vi "Main.vi"() -> ()   [LabVIEW 2020, in "RxnRover.lvlib"]
doc: "Use this template to build a simple state machine design pattern. Each state executes code and determines which state to transition to."
uses:
  RxnRover.lvlib
  RxnRover/Type Definitions/Data.ctl
  <userlib>/RxnRover/DynamicReentrant/src/Type Defs/Message.ctl
  RxnRover/Plugin Servers/Controller Array/Controller Array.lvclass
  RxnRover/Plugin Manager/Plugin Details.ctl
  RxnRover/Plugin Servers/Controller/Controller Type.ctl
  RxnRover/Plugin Manager/Plugin Types.ctl
  RxnRover/Plugin Manager/Config Error.ctl
  RxnRover/Type Definitions/New Parameters.ctl
  RxnRover/Plugin Servers/Parameter to Hardware Map/Parameter to Hardware Map.lvclass
  RxnRover/Experiment/Experiment File/Experiment File Cluster.ctl
  RxnRover/Plugin Servers/Controller/Minimal Controller Cluster.ctl
  RxnRover/Plugin Servers/Parameter to Hardware Map/Minimal Map.ctl
  RxnRover/Plugin Servers/Parameter to Hardware Map/Minimal Pair Cluster.ctl
  RxnRover/User Preferences/User Preferences File.lvclass
  RxnRover/events/Process Stopped Cluster.ctl
  RxnRover/Type Definitions/Error Levels.ctl
  RxnRover/Plugin Servers/Controller/Generic Plugin.lvclass/Generic Plugin.ctl
  RxnRover/Plugin Servers/Controller Array/Controller Array.lvclass/Controller Array.ctl
  RxnRover/Plugin Servers/Controller Array/Searchable Properties.ctl
  RxnRover/Plugin Servers/Generic Optimizer/Generic Optimizer.lvclass
  RxnRover/Sub VIs/Message Queue/Enqueue Message (Single).vi
  <vilib>/Utility/error.llb/Error Cluster From Error Code.vi
  RxnRover/Plugin Servers/Controller/Generic Plugin.lvclass
  <vilib>/ErrorRing/Error Ring.xnode
  <userlib>/RxnRover/DynamicReentrant/Dynamic Reentrant.lvlib
  RxnRover/Sub VIs/Message Queue/test Message Queue.lvlib
  RxnRover/Experiment/Experiment Manager/Experiment Manager.lvlib
  RxnRover/Experiment/Experiment File/Experiment File.lvlib
  RxnRover/Plugin Manager/Plugin Manager.lvlib
  RxnRover/logging/logging.lvlib
panel:
  in  "Stop Hardware Run Btn":bool
  in  "Start Hardware Run Btn":bool
  in  "Exit":bool
  in  "Stop Analyzer Btn":bool
  in  "Load Analyzer Btn":bool
  in  "Stop Optimizer Btn":bool
  in  "Load Optimizer Btn":bool
  in  "Stop Controller Btn":bool
  in  "Load Control Panel":bool
  in  "View an Analyzer":u16(ring) items=["None"]
  in  "Reorder Analyzers":bool
  in  "Auto Param Passing":bool=TRUE
  in  "Reassign Parameters":bool
  in  "Reject Suggestions":bool
  in  "Accept Suggestions":bool
  out "# of controllers cached":i32
  in  "Select a Plugin":u16(ring) items=["None", "Mock Temperature Controller Control Panel.lvlib:Main.vi:4140001"]
  out "# of analyzers cached":i32
  out "# of optimizers cached":i32
  out "# of plugins cached":i32
  in  "List of Running Plugins":i32(listbox)=-1
  out "Status Bar Text":string
  # "Manual Control"
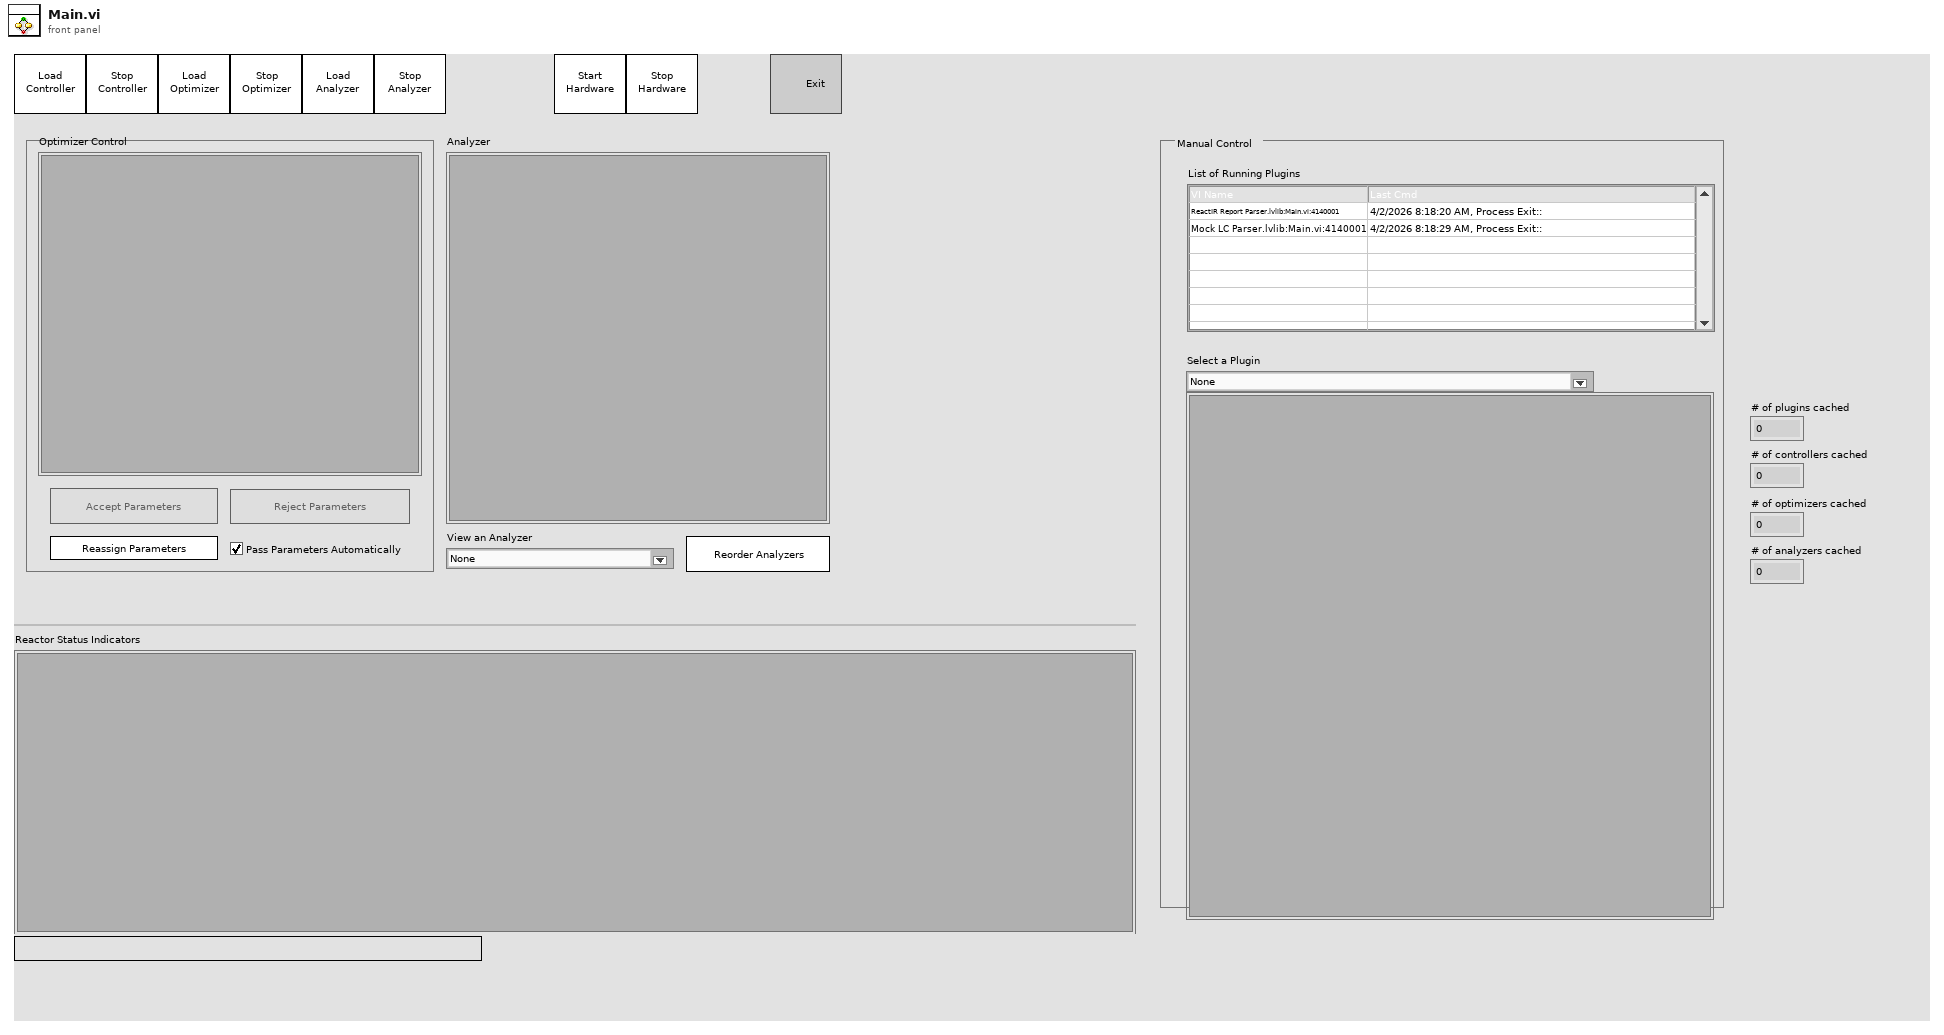
[diagram p1: front panel]
types:
  T1 = enum32{"Invalid", "Standard", "Closed", "Hidden", "Minimized", "Maximized"}
  T2 = typedef "RxnRover.lvlib/Data.ctl" = cluster{"Visible Hardware VI":string, "Current Message":T3, "Message History":string[][], "Hardware":cluster{"Process Cache":refnum<class "Controller Array.lvclass">, "Plugins":T4[]}, "Optimizers":cluster{"Process Cache":refnum<class "Controller Array.lvclass">, "Plugins":T4[], "First parameteres?":bool, "New Parameters":T8}, "Parameter to Hardware Map":refnum<class "Parameter to Hardware Map.lvclass">, "Analyzers":cluster{"Process Cache":refnum<class "Controller Array.lvclass">, "Plugins":T4[]}, "Log Directory":path, "Auto Pass Parameters":bool, "Experiment":cluster{"Name":string, "File Path":path, "File Extension":string, "File Cluster":T9}, "Main VI Queue":refnum<queue>, "Process Queue References":refnum<queue>[], "Message Queue":refnum<queue>, "User Preferences File":refnum<class "User Preferences File.lvclass">}
  T3 = typedef "Dynamic Reentrant.lvlib/Message.ctl" = cluster{"Source":string, "Destination":string, "Time Stamp":timestamp, "Command":string, "Data":variant}
  T4 = typedef "RxnRover.lvlib/Plugin Manager.lvlib/Plugin Details.ctl" = cluster{"Plugin Name":string, "Controller Type":T5, "Control Panel Path":path, "Plugin Type":T6, "Config Errors":T7[]}
  T5 = typedef "RxnRover.lvlib/Generic Plugin.lvclass/Controller Type.ctl" = enum16{"Invalid", "Temperature Controller", "Pump Controller", "Syringe Pump", "Generic Optimizer", "LC Parser", "Passive Hardware"}
  T6 = typedef "RxnRover.lvlib/Plugin Manager.lvlib/Plugin Types.ctl" = enum16{"Invalid", "Optimizer", "Analyzer", "Hardware"}
  T7 = typedef "RxnRover.lvlib/Plugin Manager.lvlib/Config Error.ctl" = cluster{"Error?":bool, "Message":string}
  T8 = typedef "RxnRover.lvlib/New Parameters.ctl" = cluster{"Time Stamp":timestamp, "Names":string[], "Values":variant[]}
  T9 = typedef "RxnRover.lvlib/Experiment File.lvlib/Experiment File Cluster.ctl" = cluster{"Hardware List":T10[], "Optimizer List":T10[], "Analyzer List":T10[], "Parameter to Hardware Map":T11}
  T10 = typedef "RxnRover.lvlib/Generic Plugin.lvclass/Minimal Controller Cluster.ctl" = cluster{"Name":string, "Controller Type":string, "Control Panel Path":string, "Resource":string}
  T11 = typedef "RxnRover.lvlib/Parameter to Hardware Map.lvclass/Minimal Map.ctl" = T12[]
  T12 = typedef "RxnRover.lvlib/Parameter to Hardware Map.lvclass/Minimal Pair Cluster.ctl" = cluster{"key":string, "values":T10[]}
  T13 = typedef "RxnRover.lvlib/Error Levels.ctl" = enum16{"Fatal", "Warning"}
  T14 = typedef "RxnRover.lvlib/Controller Array.lvclass/Searchable Properties.ctl" = enum16{"Name", "Controller Type"}
  T15 = enum8{"Enabled", "Disabled", "Disabled and Grayed Out"}
  T16 = typedef "RxnRover.lvlib/Parameter to Hardware Map.lvclass/Pair.ctl" = cluster{"key":string, "values":refnum<class "Generic Plugin.lvclass">[]}
  T17 = typedef "RxnRover.lvlib/Process Stopped Cluster.ctl" = cluster{"Name":string, "Type":enum16{"Hardware", "Optimizer", "Analyzer"}}
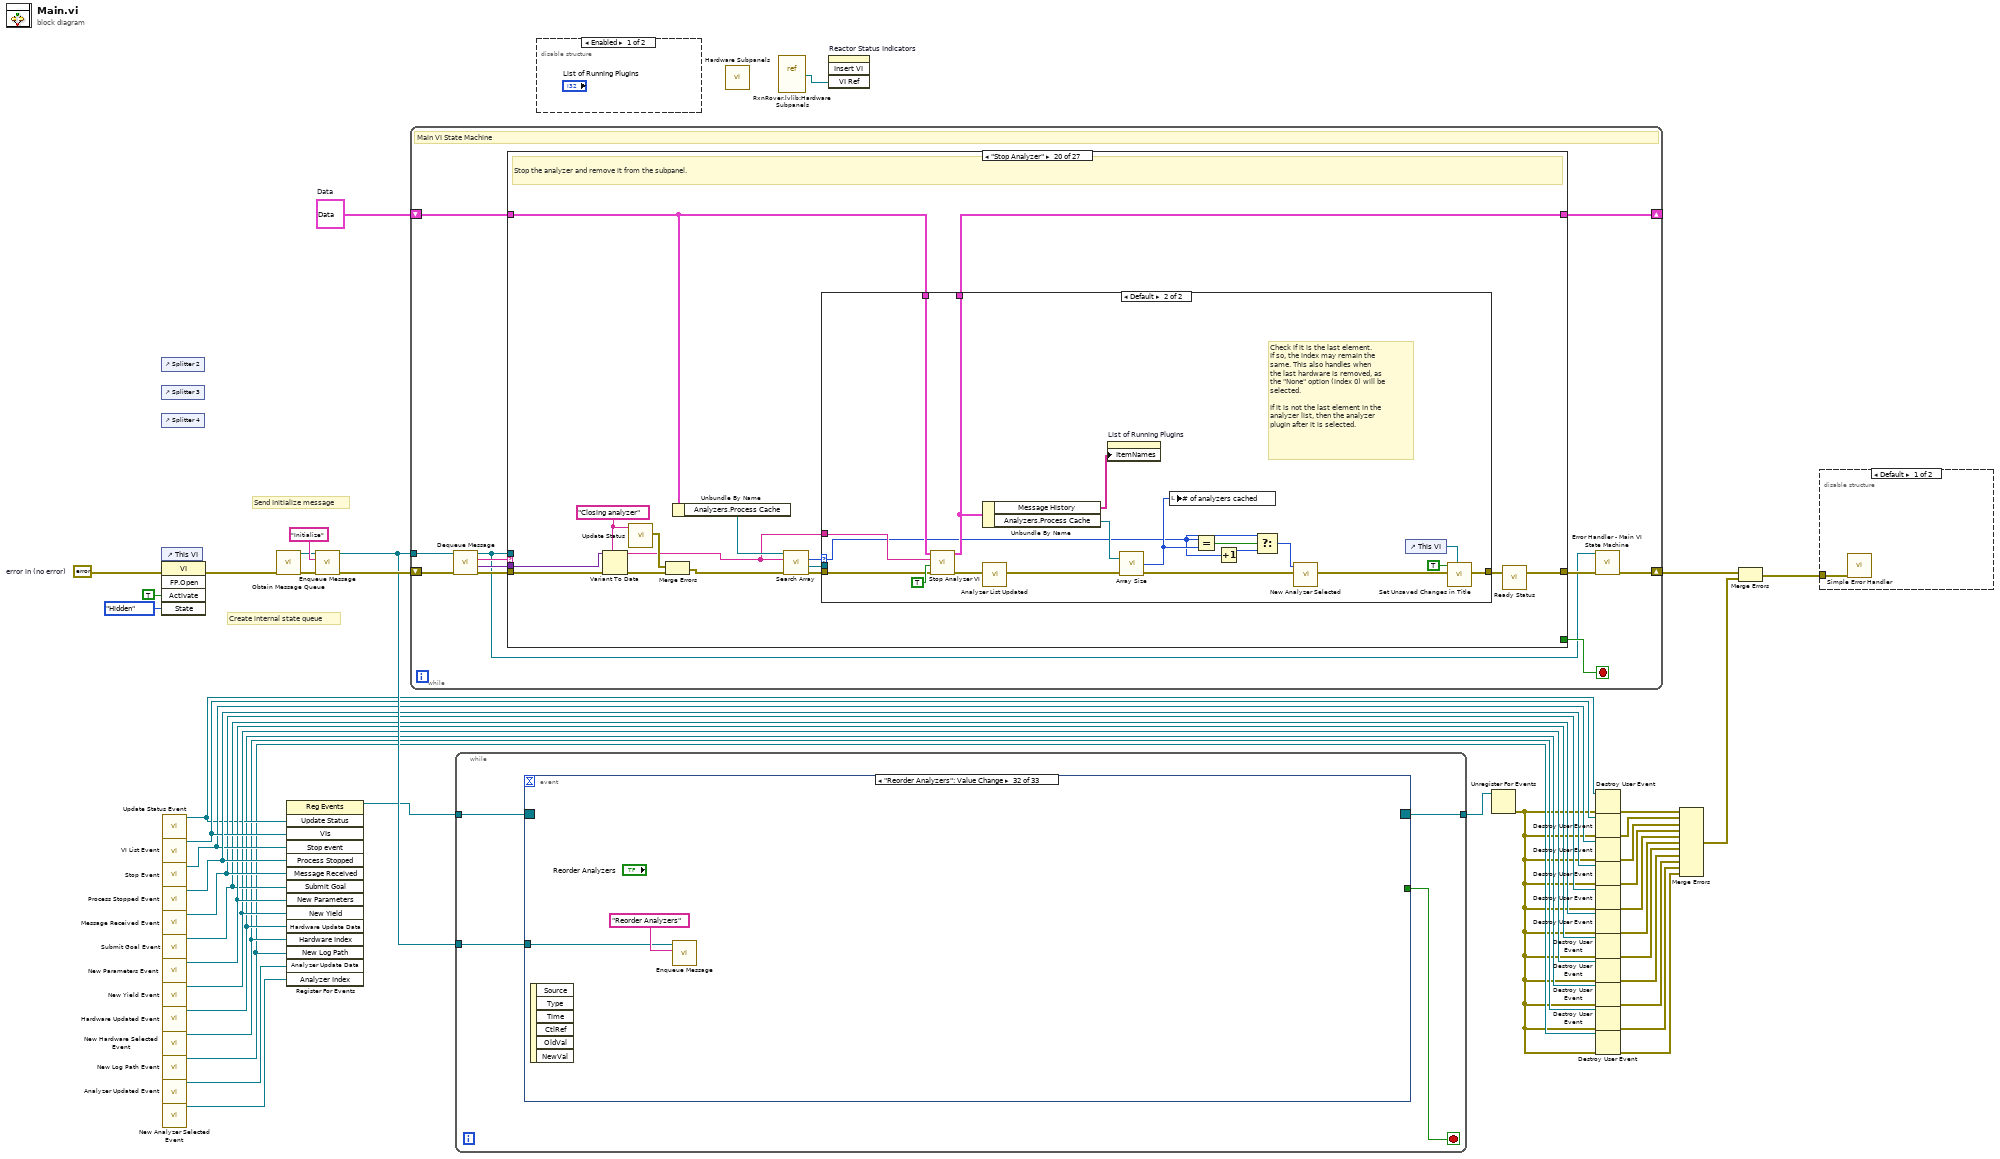
[diagram p0: block diagram]
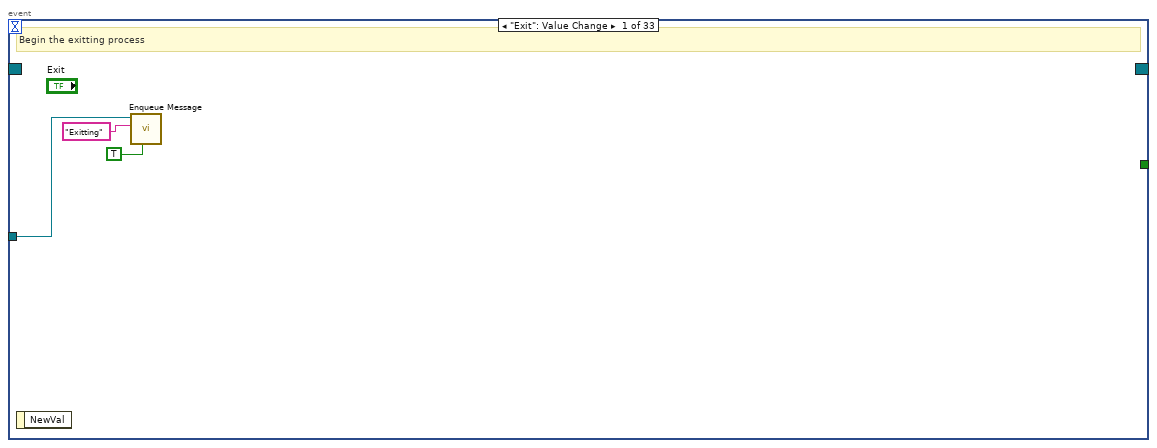
[diagram p2: hidden frame]
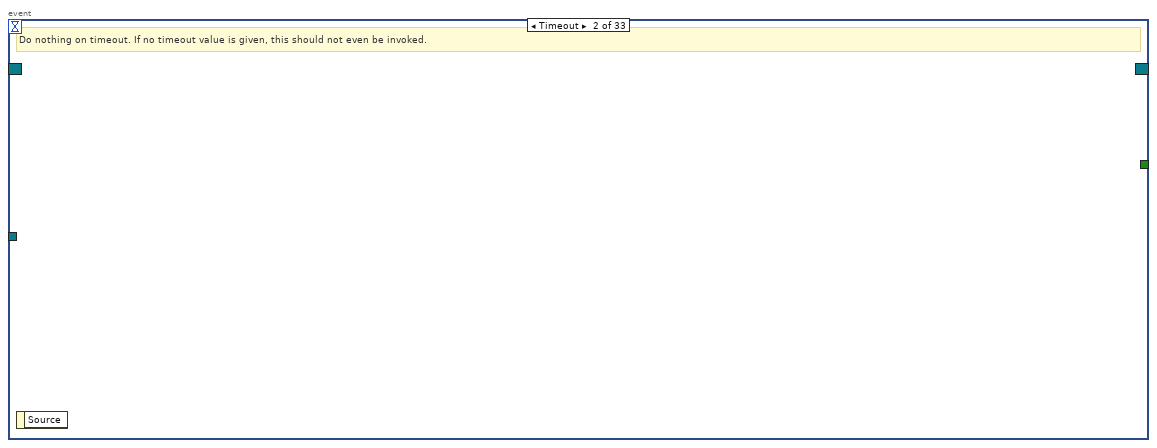
[diagram p3: hidden frame]
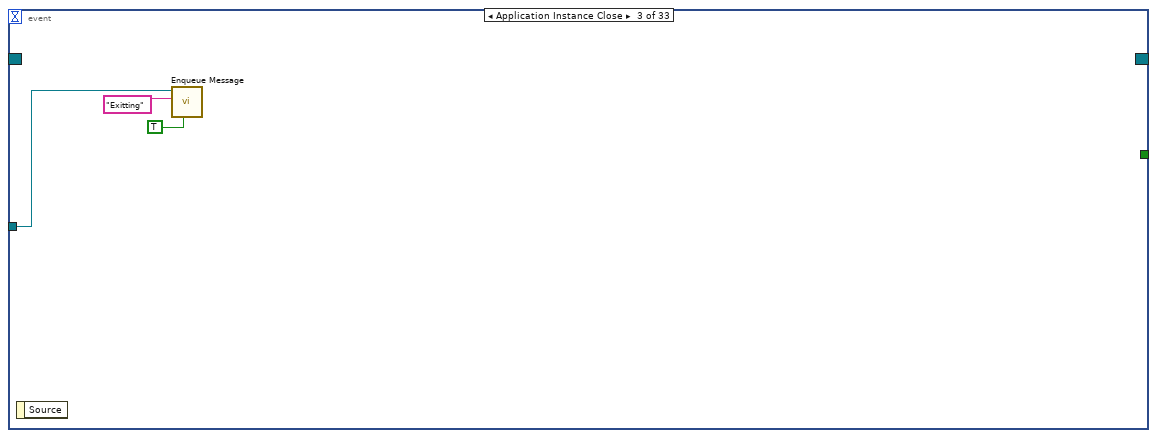
[diagram p4: hidden frame]
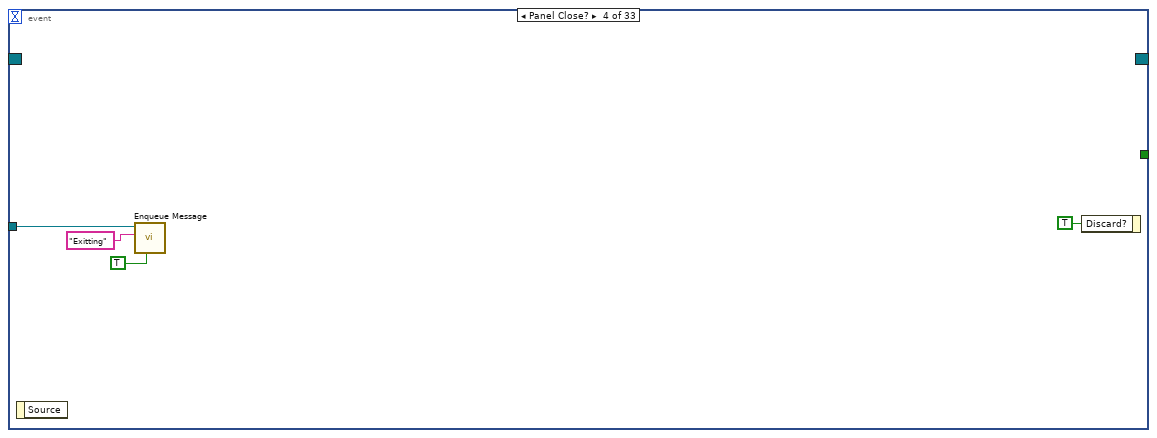
[diagram p5: hidden frame]
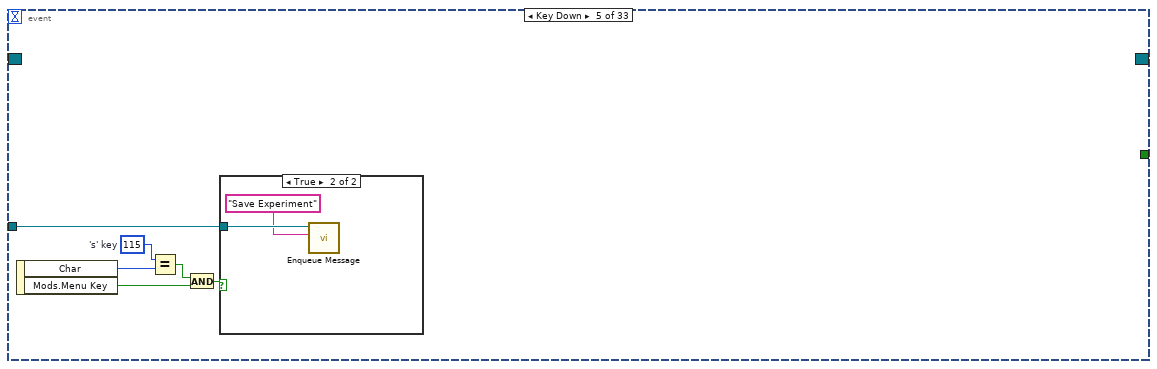
[diagram p6: hidden frame]
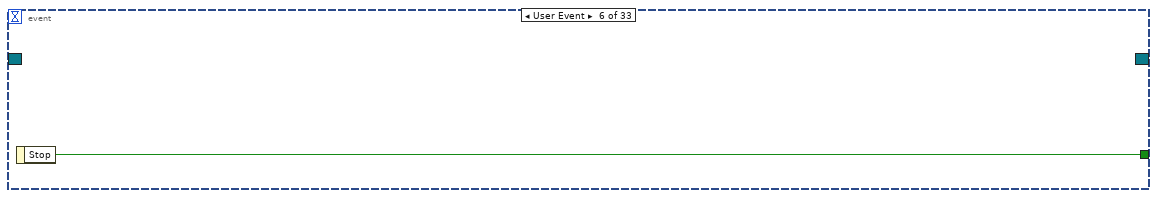
[diagram p8: hidden frame]
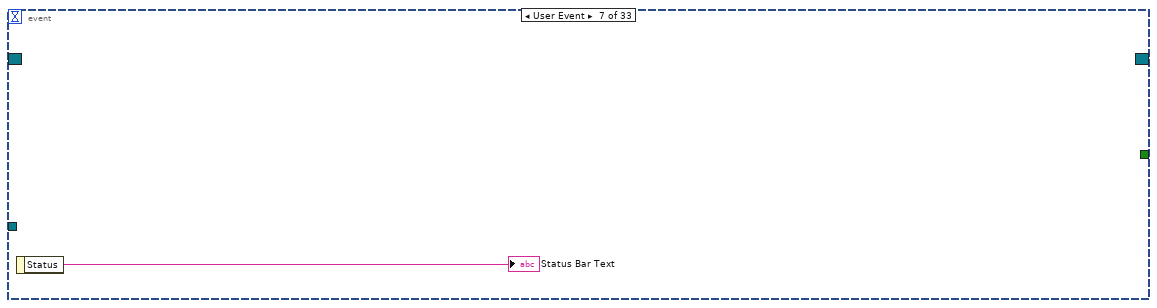
[diagram p9: hidden frame]
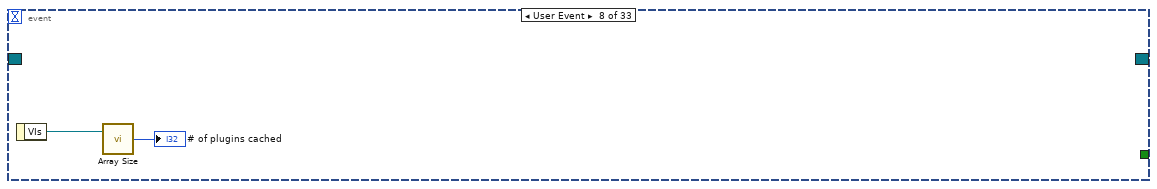
[diagram p10: hidden frame]
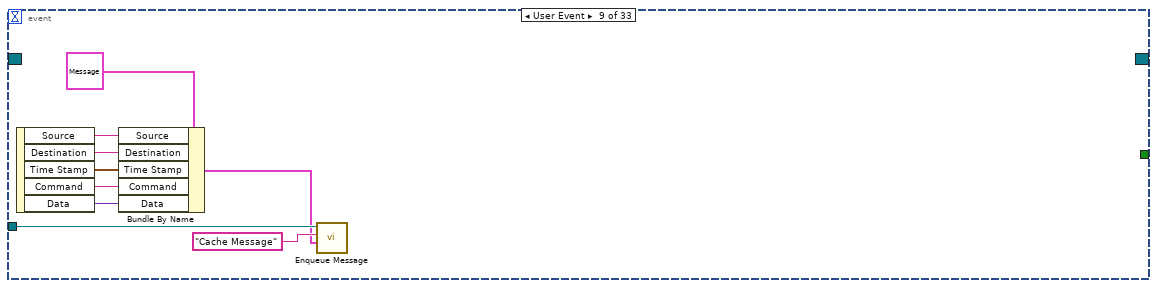
[diagram p11: hidden frame]
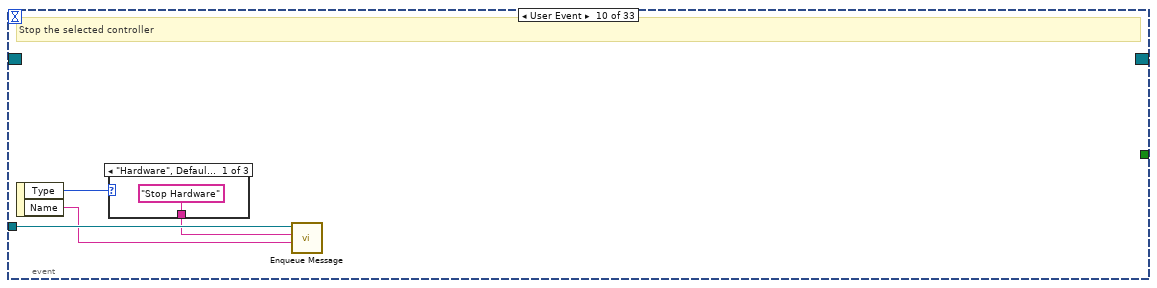
[diagram p12: hidden frame]
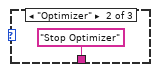
[diagram p13: hidden frame]
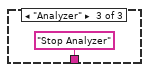
[diagram p14: hidden frame]
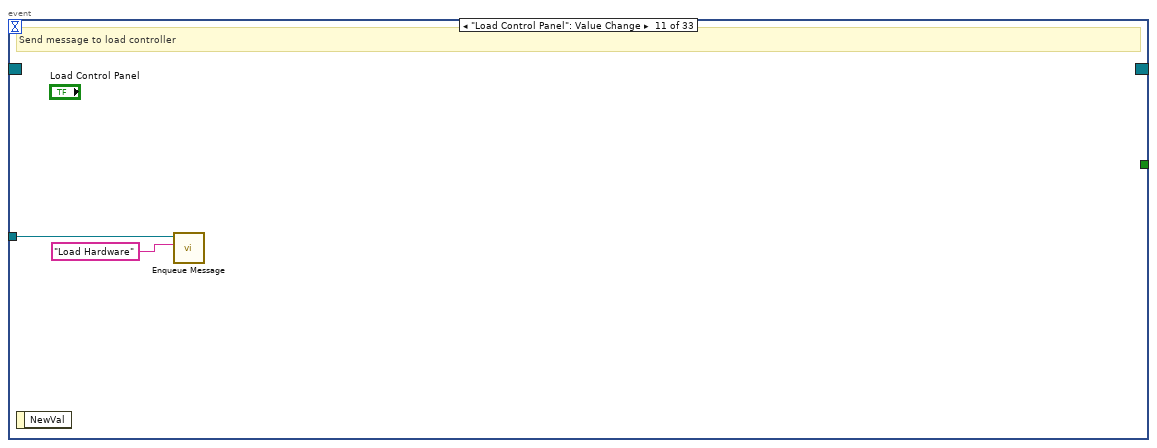
[diagram p15: hidden frame]
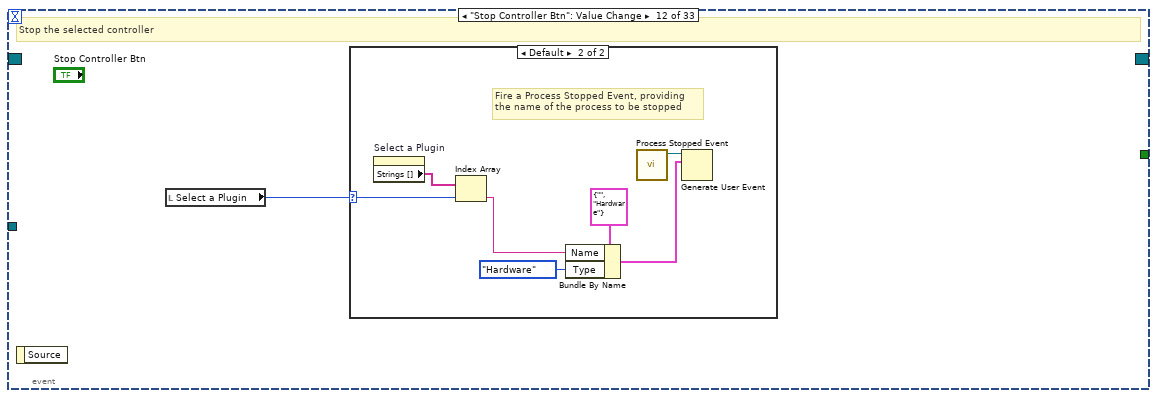
[diagram p16: hidden frame]
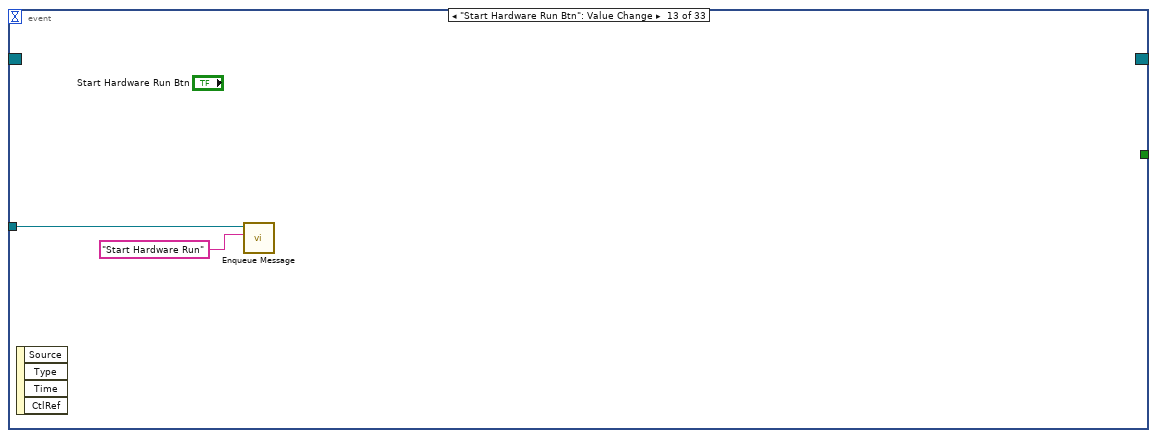
[diagram p18: hidden frame]
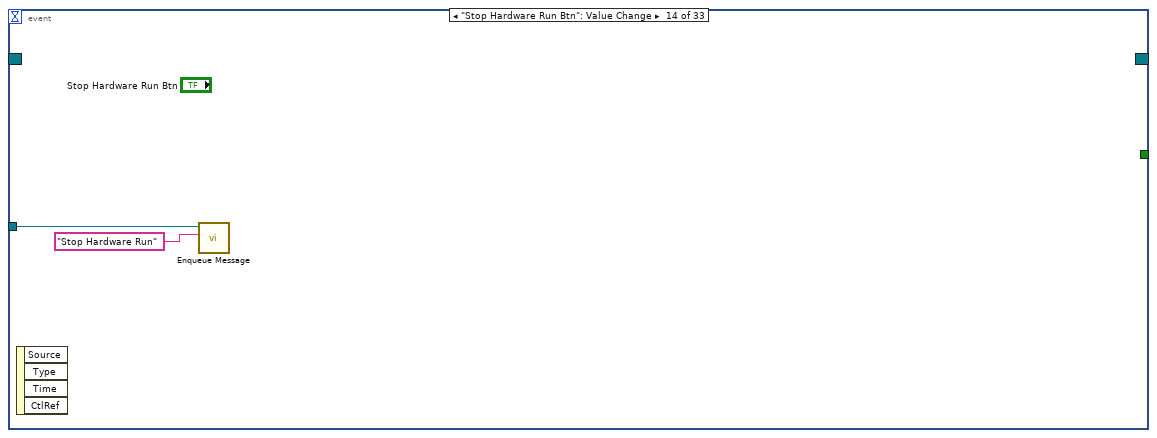
[diagram p19: hidden frame]
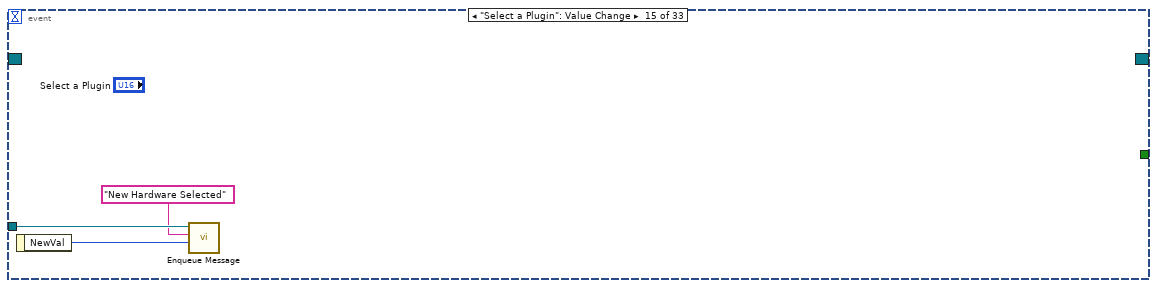
[diagram p20: hidden frame]
diagram:
  w16 = errorcluster {"status"=FALSE, "code"=0, "source"=""}  # error in (no error)
  w28 = T2 {"Visible Hardware VI"="", "Current Message"={"Source"="", "Destination"="", "Time Stamp"=timestamp(0 s since 1904-01-01), "Command"="", "Data"=variant}, "Message History"=[], "Hardware"={"Process Cache"=refnum, "Plugins"=[]}, "Optimizers"={"Process Cache"=refnum, "Plugins"=[], "First parameteres?"=FALSE, "New Parameters"={"Time Stamp"=timestamp(0 s since 1904-01-01), "Names"=[], "Values"=[]}}, "Parameter to Hardware Map"=refnum, "Analyzers"={"Process Cache"=refnum, "Plugins"=[]}, "Log Directory"=path "", "Auto Pass Parameters"=FALSE, "Experiment"={"Name"="", "File Path"=path "", "File Extension"="", "File Cluster"={"Hardware List"=[], "Optimizer List"=[], "Analyzer List"=[], "Parameter to Hardware Map"=[]}}, "Main VI Queue"=refnum, "Process Queue References"=[], "Message Queue"=refnum, "User Preferences File"=refnum}  # Data
  # "Send Initialize message"
  # "Create internal state queue"
  n1 = control-ref of="Splitter 2"() -> ()  [unwired: 1 out]
  n2 = control-ref of="Splitter 3"() -> ()  [unwired: 1 out]
  n3 = control-ref of="Splitter 4"() -> ()  [unwired: 1 out]
  n4 = control-ref of="This VI"() -> (w14:refnum<vi>)
  n5 = invoke class="VI" method="FP.Open"(reference=w14, error in=w16, "Activate"=TRUE ("Activate?"), "State"=T1."Hidden") -> (error out=w15:errorcluster)  [unwired: 1 in, 4 out]
  n6 = call "Update Status Event.vi"() -> ("Update Status"=w10:refnum<user-event>)  [unwired: 11 in]
  n7 = call "VI List Event.vi"() -> ("VIs"=w33:refnum<user-event>)  [unwired: 11 in]
  n8 = call "Stop Event.vi"() -> ("Stop event"=w27:refnum<user-event>)  [unwired: 11 out]
  n9 = call "Process Stopped Event.vi"() -> ("Process Stopped"=w34:refnum<user-event>)  [unwired: 11 in]
  n10 = call "Message Received Event.vi"() -> ("Message Received"=w25:refnum<user-event>)  [unwired: 11 in]
  n11 = call "Submit Goal Event.vi"() -> ("Submit Goal"=w23:refnum<user-event>)  [unwired: 11 in]
  n12 = call "New Parameters Event.vi"() -> ("New Parameters"=w24:refnum<user-event>)  [unwired: 11 in]
  n13 = call "New Yield Event.vi"() -> ("New Yield"=w19:refnum<user-event>)  [unwired: 11 in]
  n14 = call "Hardware Updated Event.vi"() -> ("Hardware Update Data"=w9:refnum<user-event>)  [unwired: 11 in]
  n15 = call "New Hardware Selected Event.vi"() -> ("Hardware Index"=w8:refnum<user-event>)  [unwired: 11 in]
  n16 = call "New Log Path Event.vi"() -> ("New Log Path"=w7:refnum<user-event>)  [unwired: 11 in]
  n17 = call "Analyzer Updated Event.vi"() -> ("Analyzer Update Data"=w2:refnum<user-event>)  [unwired: 11 in]
  n18 = call "New Analyzer Selected Event.vi"() -> ("Analyzer Index"=w1:refnum<user-event>)  [unwired: 11 in]
  n19 = call "Obtain Message Queue.vi"("error in (no error)"=w15) -> ("error out"=w40:errorcluster, "Message Queue"=w37:refnum<queue>)  [unwired: 9 in]
  n20 = register-events(w10, w33, w27, w34, w25, w23, w24, w19, w9, w8, w7, w2, w1) -> (reference out=w35:refnum<event-registration>)  [unwired: 2 in, 1 out]
  n21 = call-poly "Enqueue Message.vi"("error in (no error)"=w40, "Message"="Initialize", "Message Queue"=w37) -> ("error out"=w39:errorcluster, "dup Message Queue"=w36:refnum<queue>)  [unwired: 7 in]
  n22 = while {
    shift-right: [w53] -> _
    shift-left: w28 -> [w50]
    shift-right: [w44] -> w42
    shift-left: w39 -> [w52]
    tunnel: w36 -> [w48]
    stop <- w51 stop-if-true
    # "Main VI State Machine"
    n23 = call "Dequeue Message.vi"("error in (no error)"=w52, "Message Queue"=w48) -> ("error out"=w49:errorcluster, "Message Data"=w46:variant, "Message"=w47:string, "dup Message Queue"=w43:refnum<queue>)  [unwired: 6 in]
    n24 = case shown="\"Stop Analyzer\"" w47 {
      selector: w47 -> [_ _ _ _ _ _ w253 _ _ _ _ _ _ _ _ _ _ _ _ _ _ _ _ _ _ _ _]
      tunnel: [_ _ w145 w182 w243 _ _ _ _ _ _ _ _ _ _ _ _ _ _ _ _ _ _ _ _ _ _] -> w51
      tunnel: w50 -> [w70 w126 w143 w150 w239 w251 w255 w264 w281 w300 w326 w352 w372 w389 w401 w420 w467 w509 w554 w598 w640 w666 w699 w727 w756 w777 w782]
      tunnel: [w60 w126 w143 w174 w232 w252 w255 w264 w279 w300 w326 w352 w372 w389 w401 w407 w459 w499 w558 w599 w641 w653 w699 w727 w745 w775 w782] -> w53
      tunnel: w49 -> [w71 w122 w138 w175 w242 w248 _ w265 w285 w301 w327 w343 w364 w386 w398 w422 w464 w506 w566 w602 w647 w664 w707 w729 w755 w776 w785]
      tunnel: [w66 w125 w138 w181 w238 w247 w254 w263 w284 w299 w325 w342 w363 w390 w402 w418 w461 w503 w567 w601 w646 w667 w697 w724 w757 w774 w778] -> w45
      tunnel: w43 -> [w59 w120 _ w180 _ _ _ _ _ _ _ _ _ _ _ _ _ _ _ _ _ w656 _ w723 w746 _ _]
      tunnel: w46 -> [_ _ _ _ _ w249 _ _ w283 w302 w328 _ _ _ _ _ _ _ w563 w600 w645 w659 _ _ _ w773 w783]
      frame "Initialize" {
        # "Initialize - Initialize the application."
        n25 = call "Update Status.vi"("error in (no error)"=w71, "Status Bar Text"="Initializing...") -> ("error out"=w68:errorcluster)  [unwired: 9 in]
        n26 = control-ref of="This VI"() -> (w72:refnum<vi>)
        n27 = invoke class="VI" method="Default Vals.Reinit All"(reference=w72, error in=w68) -> (error out=w56:errorcluster)  [unwired: 1 in, 2 out]
        n28 = call "Load and Apply User Preferences.vi"("error in (no error)"=w56) -> ("error out"=w55:errorcluster, "User Preferences File out"=w54:refnum<class "User Preferences File.lvclass">)  [unwired: 9 in]
        n29 = call <userlib>:"Obtain Main VI Queue.vi"("error in (no error)"=w55) -> ("error out"=w61:errorcluster, "Main VI Queue"=w69:refnum<queue>)  [unwired: 9 in]
        n30 = call "Create or Load Experiment Dialog.vi"("error in (no error)"=w61, "User Preferences File.lvclass"=w54) -> ("error out"=w63:errorcluster, "Cancelled?"=w58:bool, "Experimental File Cluster"=w65:T9, "Experiment File Path"=w62:path, "Experiment File Extension"=w57:string, "Experiment Name"=w64:string)  [unwired: 4 in]
        n31 = case shown="False" w58 {
          tunnel: w70 -> [w112 w117]
          tunnel: w69 -> [w110 _]
          tunnel: [w105 errorcluster {"status"=FALSE, "code"=0, "source"=""} ("error out")] -> w66
          tunnel: w65 -> [w104 _]
          tunnel: w64 -> [w84 _]
          tunnel: w63 -> [w102 _]
          tunnel: w62 -> [w87 _]
          tunnel: [w97 w117] -> w60
          tunnel: w59 -> [_ w114]
          tunnel: w57 -> [w85 _]
          tunnel: w54 -> [w78 _]
          frame False {
            # "Show the main program window once\neverything is loaded and initialized"
            n32 = call <vilib>:"Application Directory.vi"() -> ("Application Directory"=w75:path)
            n33 = property on="Auto Param Passing" class="Bool (strict)"() -> (error out=w91:errorcluster, "Value"=w90:bool)  [unwired: 2 in, 1 out]
            n34 = control-ref of="This VI"() -> (w103:refnum<vi>)
            n35 = Format Into String(format string="Application directory: %s", w75) -> (resulting string=w73:string, error out=w74:errorcluster)  [unwired: 2 in]
            n36 = call "Update Window Title.vi"("error in (no error)"=w102, "Experiment Name"=w84, "Experiment File Path"=w87, "VI in"=w103) -> ("error out"=w101:errorcluster)  [unwired: 7 in]
            n37 = call "Log Message - DEBUG.vi"("error in (no error)"=w74, "Message"=w73) -> ()  [unwired: 9 in, 1 out]
            n38 = property on="Auto Param Passing" class="Bool (strict)"(error in=w91, "Val(Sgnl)"=w90) -> ()  [unwired: 1 in, 2 out]
            n39 = Bundle By Name(cluster=w112, "Main VI Queue"=w110, "Optimizers.First parameteres?"=TRUE ("Optimizers.First parameters?"), "User Preferences File"=w78, "Experiment.File Path"=w87, "Experiment.File Cluster"=w104, "Experiment.Name"=w84, "Experiment.File Extension"=w85, "Auto Pass Parameters"=w90) -> (w80:T2)
            n40 = Strip Path(path=w87) -> (stripped path=w88:path)  [unwired: 1 out]
            n41 = Equal?(x=w84, y="NoExperiment") -> (x = y?=w89:bool)
            n42 = Select(t=w87, s=w89, f=w88) -> (s? t:f=w86:path)
            n43 = call "Generate New Log Path Event.vi"("error in (no error)"=w101, "New Log Path"=w86) -> ("error out"=w82:errorcluster)  [unwired: 9 in]
            n44 = call "Load Details and Filter Plugins.vi"("error in (no error)"=w82, "Data in"=w80) -> ("error out"=w81:errorcluster, "Data out"=w79:T2)  [unwired: 8 in]
            n45 = call "Initialize Hardware from Experiment Cluster.vi"("error in (no error)"=w81, "Reaction Rover Data"=w79) -> ("error out"=w96:errorcluster, "Reaction Rover Data out"=w94:T2)  [unwired: 7 in, 1 out]
            n46 = call "Initialize Parameter to Hardware Map from Experiment Cluster.vi"("error in (no error)"=w96, "Reaction Rover Data in"=w94) -> ("error out"=w95:errorcluster, "Reaction Rover Data out"=w93:T2)  [unwired: 8 in]
            n47 = control-ref of="Optimizer Control"() -> (w92:refnum<vi>)
            n48 = call "Initialize Optimizer from Experiment Cluster.vi"("Optimizer Control"=w92, "error in (no error)"=w95, "Reaction Rover Data"=w93) -> ("error out"=w100:errorcluster, "Reaction Rover Data out"=w98:T2)  [unwired: 6 in, 1 out]
            n49 = call "Initialize Analyzer from Experiment Cluster.vi"("error in (no error)"=w100, "Reaction Rover Data"=w98) -> ("error out"=w99:errorcluster, "Reaction Rover Data out"=w97:T2)  [unwired: 7 in, 1 out]
            n50 = control-ref of="This VI"() -> (w108:refnum<vi>)
            n51 = invoke class="VI" method="FP.Open"(reference=w108, error in=w99, "Activate"=TRUE ("Activate?"), "State"=T1."Maximized") -> (error out=w109:errorcluster)  [unwired: 1 in, 4 out]
            n52 = property on="List of Running Plugins" class="MCListbox (strict)"("ItemNames"=string[][] [] ("Item Names")) -> ()  [unwired: 2 in, 2 out]
            n53 = call "Ready Status.vi"("error in (no error)"=w109) -> ("error out"=w105:errorcluster)  [unwired: 2 in]
          }
          frame True {
            # "Close the application if the experiment selector was cancelled."
            n54 = call-poly "Enqueue Message.vi"("Priority Message? (F)"=TRUE, "Message"="Exit", "Message Queue"=w114) -> ()  [unwired: 7 in, 2 out]
          }
        }
      }
      frame "Error" {
        # "Handle errors and warnings, determining if the error warrants program shutdown."
        n55 = call "Update Status.vi"("error in (no error)"=w122, "Status Bar Text"="Error!") -> ("error out"=w119:errorcluster)  [unwired: 9 in]
        n56 = Unbundle By Name(w119) -> ("code"=w124:i32)
        n57 = Less Than 0?(x=w124) -> (x < 0?=w123:bool)
        n58 = case shown="True" w123 {
          tunnel: [Error_Levels."Warning" Error_Levels."Fatal"] -> w121
          frame False {
          }
          frame True {
          }
        }
        n59 = case shown="\"Fatal\", Default" w121 {
          tunnel: [w130 w133] -> w125
          tunnel: w119 -> [w131 w135]
          tunnel: w120 -> [w129 _]
          frame "Fatal", Default {
            n60 = call <vilib>:"Simple Error Handler.vi"("error in (no error)"=w131) -> ("error out"=w132:errorcluster)  [unwired: 4 in, 4 out]
            n61 = call <vilib>:"Clear Errors.vi"("error in (no error)"=w132) -> ("error out"=w127:errorcluster)  [unwired: 5 in, 1 out]
            n62 = call-poly "Enqueue Message.vi"("error in (no error)"=w127, "Message"="Exitting", "Message Queue"=w129) -> ("error out"=w130:errorcluster)  [unwired: 7 in, 1 out]
          }
          frame "Warning" {
            n63 = call <vilib>:"Simple Error Handler.vi"("error in (no error)"=w135) -> ("error out"=w134:errorcluster)  [unwired: 4 in, 4 out]
            n64 = call <vilib>:"Clear Errors.vi"("error in (no error)"=w134) -> ("error out"=w133:errorcluster)  [unwired: 5 in, 1 out]
          }
        }
      }
      frame "Exit" {
        w139 = TRUE  # Stop
        w145 = TRUE  # Stop Loop?
        # "Release these queue references in a delayed way. We do not want to release them before the process VI has received the message."
        # "Exit - Exit the application."
        n65 = call "Stop Event.vi"() -> ("Stop event"=w141:refnum<user-event>)  [unwired: 11 out]
        n66 = Generate User Event(user event=w141, event data cluster=w139) -> (error out=w140:errorcluster)  [unwired: 2 in, 1 out]
        n67 = call <vilib>:"Simple Error Handler.vi"("error in (no error)"=w140) -> ()  [unwired: 4 in, 5 out]
        n68 = Unbundle By Name(w143) -> ("Process Queue References"=w144:refnum<queue>[], "Main VI Queue"=w142:refnum<queue>)
        n69 = for {
          tunnel: w144 -> [w146] mode=indexing
          n70 = Release Queue(queue=w146) -> ()  [unwired: 2 in, 3 out]
        }
        n71 = Release Queue(queue=w142) -> ()  [unwired: 2 in, 3 out]
      }
      frame "Exitting" {
        w181 = errorcluster {"status"=FALSE, "code"=0, "source"=""}  # error out
        w182 = FALSE  # Stop Loop?
        # "Make sure each hardware has been\ninstructed to stop before attempting\nto shut down the controllers"
        # "Send Exit Command to all open Process VIs. Doing a Force Destroy on all the queues of the process VIs will also have the same effect, based on how the process VI is currently written."
        # "Errors need to be shown here or they will be ignored since there is no room to enter the Error state anymore."
        # "Start at the back of the array"
        # "Begin exitting the application"
        n72 = Unbundle By Name(w150) -> ("Optimizers.Process Cache"=w172:refnum<class "Controller Array.lvclass">)
        n73 = call "Update Status.vi"("error in (no error)"=w175, "Status Bar Text"="Exitting") -> ("error out"=w152:errorcluster)  [unwired: 9 in]
        n74 = call "Save Reaction Rover Data to Experiment File.vi"("error in (no error)"=w152, "Reaction Rover Data"=w150) -> ("error out"=w151:errorcluster)  [unwired: 7 in, 2 out]
        n75 = call "Array Size.vi"("Controller Array in"=w172, "error in (no error)"=w151) -> ("Controller Array out"=w167:refnum<class "Controller Array.lvclass">, "size(s)"=w168:i32, "error out"=w169:errorcluster)
        n76 = Decrement(x=w168) -> (x-1=w166:i32)
        n77 = for {
          N: w168 -> [_]
          shift-right: [w202] -> w158
          shift-left: w169 -> [w215]
          tunnel: w166 -> [w210]
          tunnel: w167 -> [w209]
          shift-right: [w201] -> w160
          shift-left: w150 -> [w204]
          i -> [w211]
          n78 = Subtract(x=w210, y=w211) -> (x-y=w212:i32)
          n79 = call "Index Array.vi"("error in (no error)"=w215, "index"=w212, "Controller Array in"=w209) -> ("error out"=w213:errorcluster, "element"=w208:refnum<class "Generic Plugin.lvclass">)  [unwired: 1 out]
          n80 = call "Read Name.vi"("controller in"=w208, "error in (no error)"=w213) -> ("Name"=w206:string, "error out"=w207:errorcluster)  [unwired: 1 out]
          n81 = call "Stop Optimizer VI.vi"("error in (no error)"=w207, "Blocking (T)"=TRUE, "Process Name"=w206, "Data in"=w204) -> ("error out"=w203:errorcluster, "Data out"=w201:T2)  [unwired: 6 in]
          n82 = Unbundle By Name(w201) -> ("Message History"=w205:string[][])
          n83 = invoke on="Optimizer Control" class="SubPnl" method="Remove VI"(error in=w203) -> (error out=w202:errorcluster)  [unwired: 2 in, 2 out]
          n84 = property on="List of Running Plugins" class="MCListbox (strict)"("ItemNames"=w205) -> ()  [unwired: 2 in, 2 out]
        }
        n85 = Unbundle By Name(w160) -> ("Analyzers.Process Cache"=w161:refnum<class "Controller Array.lvclass">)
        n86 = call "Array Size.vi"("Controller Array in"=w161, "error in (no error)"=w158) -> ("Controller Array out"=w164:refnum<class "Controller Array.lvclass">, "size(s)"=w163:i32, "error out"=w162:errorcluster)
        n87 = Decrement(x=w163) -> (x-1=w165:i32)
        n88 = for {
          N: w163 -> [_]
          shift-right: [w187] -> w156
          shift-left: w162 -> [w200]
          tunnel: w165 -> [w195]
          tunnel: w164 -> [w194]
          shift-right: [w186] -> w159
          shift-left: w160 -> [w189]
          i -> [w196]
          n89 = Subtract(x=w195, y=w196) -> (x-y=w197:i32)
          n90 = call "Index Array.vi"("error in (no error)"=w200, "index"=w197, "Controller Array in"=w194) -> ("error out"=w198:errorcluster, "element"=w193:refnum<class "Generic Plugin.lvclass">)  [unwired: 1 out]
          n91 = call "Read Name.vi"("controller in"=w193, "error in (no error)"=w198) -> ("Name"=w191:string, "error out"=w192:errorcluster)  [unwired: 1 out]
          n92 = call "Stop Analyzer VI.vi"("error in (no error)"=w192, "Blocking (T)"=TRUE, "Process Name"=w191, "Data in"=w189) -> ("error out"=w188:errorcluster, "Data out"=w186:T2)  [unwired: 6 in]
          n93 = Unbundle By Name(w186) -> ("Message History"=w190:string[][])
          n94 = invoke on="Analyzer" class="SubPnl" method="Remove VI"(error in=w188) -> (error out=w187:errorcluster)  [unwired: 2 in, 2 out]
          n95 = property on="List of Running Plugins" class="MCListbox (strict)"("ItemNames"=w190) -> ()  [unwired: 2 in, 2 out]
        }
        n96 = Unbundle By Name(w159) -> ("Hardware.Process Cache"=w157:refnum<class "Controller Array.lvclass">)
        n97 = call "Read Array.vi"("error in (no error)"=w156, "Controller Array in"=w157) -> ("error out"=w154:errorcluster, "Array"=w155:refnum<class "Generic Plugin.lvclass">[])  [unwired: 7 in, 1 out]
        n98 = for {
          tunnel: w155 -> [w185] mode=indexing
          shift-right: [w183] -> w153
          shift-left: w154 -> [w184]
          n99 = call "Send Stop Message.vi"("error in (no error)"=w184, "Generic Controller in"=w185) -> ("error out"=w183:errorcluster)  [unwired: 8 in, 1 out]
        }
        n100 = call "Array Size.vi"("Controller Array in"=w157, "error in (no error)"=w153) -> ("Controller Array out"=w171:refnum<class "Controller Array.lvclass">, "size(s)"=w178:i32, "error out"=w170:errorcluster)
        n101 = Decrement(x=w178) -> (x-1=w177:i32)
        n102 = for {
          N: w178 -> [_]
          shift-right: [w218] -> w148
          shift-left: w170 -> [w229]
          tunnel: w177 -> [w225]
          shift-right: [w220] -> w174
          shift-left: w159 -> [w221]
          tunnel: w171 -> [w222]
          i -> [w224]
          n103 = Subtract(x=w225, y=w224) -> (x-y=w223:i32)
          n104 = call "Index Array.vi"("error in (no error)"=w229, "index"=w223, "Controller Array in"=w222) -> ("error out"=w227:errorcluster, "element"=w228:refnum<class "Generic Plugin.lvclass">)  [unwired: 1 out]
          n105 = call "Read Name.vi"("controller in"=w228, "error in (no error)"=w227) -> ("Name"=w217:string, "error out"=w226:errorcluster)  [unwired: 1 out]
          n106 = call "Stop Process VI.vi"("error in (no error)"=w226, "Blocking (T)"=TRUE, "Process Name"=w217, "Data in"=w221) -> ("error out"=w218:errorcluster, "Data out"=w220:T2)  [unwired: 6 in]
          n107 = Unbundle By Name(w220) -> ("Message History"=w219:string[][])
          n108 = property on="List of Running Plugins" class="MCListbox (strict)"("ItemNames"=w219) -> ()  [unwired: 2 in, 2 out]
        }
        n109 = invoke on="Selected Plugin" class="SubPnl" method="Remove VI"(error in=w148) -> (error out=w147:errorcluster)  [unwired: 2 in, 2 out]
        n110 = call <vilib>:"Clear Errors.vi"("error in (no error)"=w147) -> ("error out"=w149:errorcluster)  [unwired: 5 in, 1 out]
        n111 = call-poly "Enqueue Message.vi"("Priority Message? (F)"=TRUE, "error in (no error)"=w149, "Message"="Exit", "Message Queue"=w180) -> ()  [unwired: 6 in, 2 out]
        n112 = call <vilib>:"Simple Error Handler.vi"("error in (no error)"=w147) -> ()  [unwired: 4 in, 5 out]
      }
      frame "Save Experiment" {
        w243 = FALSE  # Stop Loop?
        # "Save the current state to the experiment file."
        n113 = call "Update Status.vi"("error in (no error)"=w242, "Status Bar Text"="Saving...") -> ("error out"=w240:errorcluster)  [unwired: 9 in]
        n114 = call "Save Reaction Rover Data to Experiment File.vi"("error in (no error)"=w240, "Reaction Rover Data"=w239) -> ("error out"=w235:errorcluster, "Reaction Rover Data out"=w232:T2)  [unwired: 7 in, 1 out]
        n115 = Unbundle By Name(w232) -> ("Experiment.File Path"=w231:path, "Experiment.Name"=w230:string)
        n116 = control-ref of="This VI"() -> (w233:refnum<vi>)
        n117 = call "Update Window Title.vi"("error in (no error)"=w235, "Experiment Name"=w230, "Experiment File Path"=w231, "VI in"=w233) -> ("error out"=w234:errorcluster)  [unwired: 7 in]
        n118 = call "Set Unsaved Changes in Title.vi"("VI in"=w233, "error in (no error)"=w234, "Unsaved changes? (F)"=FALSE) -> ("error out"=w237:errorcluster)  [unwired: 8 in]
        n119 = call "Ready Status.vi"("error in (no error)"=w237) -> ("error out"=w238:errorcluster)  [unwired: 2 in]
      }
      frame "Cache Message" {
        # "Always cache the message in the history"
        n120 = Variant To Data(error in=w248, type=T3 {"Source"="", "Destination"="", "Time Stamp"=timestamp(0 s since 1904-01-01), "Command"="", "Data"=variant} ("Message"), Variant=w249) -> (data=w246:T3, error out=w247:errorcluster)
        n121 = Unbundle By Name(w251) -> ("Message History"=w244:string[][])
        n122 = call "Cache Message.vi"("Message"=w246, "Message History In"=w244) -> ("Message History Out"=w245:string[][])  [unwired: 9 in]
        n123 = property on="List of Running Plugins" class="MCListbox (strict)"("ItemNames"=w245) -> ()  [unwired: 2 in, 2 out]
        n124 = Bundle By Name(cluster=w251, "Message History"=w245) -> (w252:T2)
      }
      frame Default {
        n125 = xnode "Error Ring"("parameter 0"=w253) -> ("error out"=w254:errorcluster)
      }
      frame "--- Copy this Frame ---" {
        n126 = call "Ready Status.vi"("error in (no error)"=w265) -> ("error out"=w263:errorcluster)  [unwired: 2 in]
      }
      frame "New Log Path" {
        # "Send the new log directory to all plugins"
        # "Update the logging directory."
        n127 = Variant To Data(error in=w285, type=path "", Variant=w283) -> (data=w280:path, error out=w277:errorcluster)
        n128 = Bundle By Name(cluster=w281, "Log Directory"=w280) -> (w279:T2)
        n129 = Unbundle By Name(w279) -> ("Log Directory"=w275:path, "Optimizers.Process Cache"=w266:refnum<class "Controller Array.lvclass">, "Analyzers.Process Cache"=w267:refnum<class "Controller Array.lvclass">, "Hardware.Process Cache"=w278:refnum<class "Controller Array.lvclass">)
        n130 = call "Read Array.vi"("error in (no error)"=w277, "Controller Array in"=w278) -> ("error out"=w274:errorcluster, "Array"=w268:refnum<class "Generic Plugin.lvclass">[])  [unwired: 7 in, 1 out]
        n131 = call "Read Array.vi"("error in (no error)"=w274, "Controller Array in"=w267) -> ("error out"=w273:errorcluster, "Array"=w269:refnum<class "Generic Plugin.lvclass">[])  [unwired: 7 in, 1 out]
        n132 = call "Read Array.vi"("error in (no error)"=w273, "Controller Array in"=w266) -> ("error out"=w272:errorcluster, "Array"=w270:refnum<class "Generic Plugin.lvclass">[])  [unwired: 7 in, 1 out]
        n133 = Build Array (concatenate)(w268, w269, w270) -> (w271:refnum<class "Generic Plugin.lvclass">[])
        n134 = for {
          tunnel: w272 -> [w289]
          tunnel: w271 -> [w288] mode=indexing
          tunnel: [w287] -> w276
          tunnel: w275 -> [w286]
          n135 = call "Send Log Directory Message.vi"("error in (no error)"=w289, "Log Directory"=w286, "Generic Controller in"=w288) -> ("error out"=w287:errorcluster)  [unwired: 7 in, 1 out]
        }
        n136 = call "Ready Status.vi"("error in (no error)"=w276) -> ("error out"=w284:errorcluster)  [unwired: 2 in]
      }
      frame "New Hardware Selected" {
        # "Update the currently visible hardware control panel"
        n137 = Variant To Data(error in=w301, type=u16 0, Variant=w302) -> (data=w290:u16, error out=w298:errorcluster)
        n138 = Unbundle By Name(w300) -> ("Hardware.Process Cache"=w292:refnum<class "Controller Array.lvclass">)
        n139 = Less Or Equal To 0?(x=w290) -> (x <= 0?=w293:bool)
        n140 = call "Array Size.vi"("Controller Array in"=w292, "error in (no error)"=w298) -> ("size(s)"=w294:i32, "error out"=w297:errorcluster)  [unwired: 1 out]
        n141 = Greater?(x=w290, y=w294) -> (0:w295:bool)
        n142 = Or(x=w293, y=w295) -> (x .or. y?=w296:bool)
        n143 = case shown="True" w296 {
          tunnel: w297 -> [w312 w315]
          tunnel: [w309 w314] -> w299
          tunnel: w290 -> [w307 _]
          tunnel: w292 -> [w306 _]
          tunnel: [w305 w313] -> w291
          tunnel: w290 -> [w305 _]
          frame False {
            # "Load the new plugin front panel."
            n144 = Decrement(x=w307) -> (x-1=w308:u16)
            n145 = call "Index Array.vi"("error in (no error)"=w312, "index"=w308, "Controller Array in"=w306) -> ("error out"=w311:errorcluster, "element"=w310:refnum<class "Generic Plugin.lvclass">)  [unwired: 1 out]
            n146 = control-ref of="Selected Plugin"() -> (w304:refnum<vi>)
            n147 = call "Load Plugin Front Panel.vi"("error in (no error)"=w311, "Sub Panel"=w304, "Generic Controller in"=w310) -> ("error out"=w309:errorcluster)  [unwired: 8 in]
          }
          frame True {
            w313 = u16 0 items=["None", "Mock Pump Controller.lvlib:Main.vi:4140003"] ("Select a Plugin")
            # "Remove any VI present since either \"None\" or an invalid index was given, which could be negative or higher than the max index."
            n148 = invoke on="Selected Plugin" class="SubPnl" method="Remove VI"(error in=w315) -> (error out=w314:errorcluster)  [unwired: 2 in, 2 out]
          }
        }
        n149 = local write "Select a Plugin"(w291) -> ()
      }
      frame "New Analyzer Selected" {
        # "Update the currently visible analyzer control panel"
        n150 = Unbundle By Name(w326) -> ("Analyzers.Process Cache"=w318:refnum<class "Controller Array.lvclass">)
        n151 = Variant To Data(error in=w327, type=u16 0, Variant=w328) -> (data=w316:u16, error out=w324:errorcluster)
        n152 = Less Or Equal To 0?(x=w316) -> (x <= 0?=w319:bool)
        n153 = call "Array Size.vi"("Controller Array in"=w318, "error in (no error)"=w324) -> ("size(s)"=w320:i32, "error out"=w323:errorcluster)  [unwired: 1 out]
        n154 = Greater?(x=w316, y=w320) -> (0:w321:bool)
        n155 = Or(x=w319, y=w321) -> (x .or. y?=w322:bool)
        n156 = case shown="False" w322 {
          tunnel: w323 -> [w338 w341]
          tunnel: [w335 w340] -> w325
          tunnel: w316 -> [w333 _]
          tunnel: w318 -> [w332 _]
          tunnel: [w331 w339] -> w317
          tunnel: w316 -> [w331 _]
          frame False {
            # "Load the new plugin front panel."
            n157 = Decrement(x=w333) -> (x-1=w334:u16)
            n158 = call "Index Array.vi"("error in (no error)"=w338, "index"=w334, "Controller Array in"=w332) -> ("error out"=w337:errorcluster, "element"=w336:refnum<class "Generic Plugin.lvclass">)  [unwired: 1 out]
            n159 = control-ref of="Analyzer"() -> (w330:refnum<vi>)
            n160 = call "Load Plugin Front Panel.vi"("error in (no error)"=w337, "Sub Panel"=w330, "Generic Controller in"=w336) -> ("error out"=w335:errorcluster)  [unwired: 8 in]
          }
          frame True {
            w339 = u16 0 items=["None", "Mock Pump Controller.lvlib:Main.vi:4140003"] ("Select a Plugin")
            # "Remove any VI present since either \"None\" or an invalid index was given, which could be negative or higher than the max index."
            n161 = invoke on="Analyzer" class="SubPnl" method="Remove VI"(error in=w341) -> (error out=w340:errorcluster)  [unwired: 2 in, 2 out]
          }
        }
        n162 = local write "View an Analyzer"(w317) -> ()
      }
      frame "Refresh Hardware Selector" {
        # "Loop over all hardware processes and get their names"
        # "Refreshes the list of harware the user can select for manual control."
        n163 = Unbundle By Name(w352) -> ("Hardware.Process Cache"=w351:refnum<class "Controller Array.lvclass">)
        n164 = call "Array Size.vi"("Controller Array in"=w351, "error in (no error)"=w343) -> ("Controller Array out"=w350:refnum<class "Controller Array.lvclass">, "size(s)"=w348:i32, "error out"=w349:errorcluster)
        n165 = for {
          N: w348 -> [_]
          tunnel: w350 -> [w361]
          shift-right: [w357] -> w344
          shift-left: w349 -> [w359]
          shift-right: [w355] -> w345
          shift-left: string[] ["None"] -> [w356]
          i -> [w360]
          n166 = call "Index Array.vi"("error in (no error)"=w359, "index"=w360, "Controller Array in"=w361) -> ("error out"=w358:errorcluster, "element"=w353:refnum<class "Generic Plugin.lvclass">)  [unwired: 1 out]
          n167 = call "Read Name.vi"("controller in"=w353, "error in (no error)"=w358) -> ("Name"=w354:string, "error out"=w357:errorcluster)  [unwired: 1 out]
          n168 = Build Array (concatenate)(w356, w354) -> (w355:string[])
        }
        n169 = control-ref of="Select a Plugin"() -> (w346:refnum<vi>)
        n170 = property class="Ring (strict)"(reference=w346, error in=w344, "Strings []"=w345) -> (error out=w342:errorcluster)  [unwired: 1 out]
      }
      frame "Refresh Analyzer Selector" {
        # "Loop over all analyzer processes and get their names"
        # "Refreshes the list of analyzers the user can select to view."
        n171 = Unbundle By Name(w372) -> ("Analyzers.Process Cache"=w371:refnum<class "Controller Array.lvclass">)
        n172 = call "Array Size.vi"("Controller Array in"=w371, "error in (no error)"=w364) -> ("Controller Array out"=w370:refnum<class "Controller Array.lvclass">, "size(s)"=w368:i32, "error out"=w369:errorcluster)
        n173 = for {
          N: w368 -> [_]
          tunnel: w370 -> [w381]
          shift-right: [w377] -> w365
          shift-left: w369 -> [w379]
          shift-right: [w375] -> w366
          shift-left: string[] ["None"] -> [w376]
          i -> [w380]
          n174 = call "Index Array.vi"("error in (no error)"=w379, "index"=w380, "Controller Array in"=w381) -> ("error out"=w378:errorcluster, "element"=w373:refnum<class "Generic Plugin.lvclass">)  [unwired: 1 out]
          n175 = call "Read Name.vi"("controller in"=w373, "error in (no error)"=w378) -> ("Name"=w374:string, "error out"=w377:errorcluster)  [unwired: 1 out]
          n176 = Build Array (concatenate)(w376, w374) -> (w375:string[])
        }
        n177 = control-ref of="View an Analyzer"() -> (w362:refnum<vi>)
        n178 = property class="Ring (strict)"(reference=w362, error in=w365, "Strings []"=w366) -> (error out=w363:errorcluster)  [unwired: 1 out]
      }
      frame "Start Hardware Run" {
        n179 = Unbundle By Name(w389) -> ("Hardware.Process Cache"=w388:refnum<class "Controller Array.lvclass">)
        n180 = call "Update Status.vi"("error in (no error)"=w386, "Status Bar Text"="Starting hardware run.") -> ("error out"=w383:errorcluster)  [unwired: 9 in]
        n181 = call "Read Array.vi"("error in (no error)"=w383, "Controller Array in"=w388) -> ("error out"=w385:errorcluster, "Array"=w387:refnum<class "Generic Plugin.lvclass">[])  [unwired: 7 in, 1 out]
        n182 = for {
          tunnel: w387 -> [w392] mode=indexing
          shift-right: [w391] -> w384
          shift-left: w385 -> [w393]
          n183 = call "Send Start Message.vi"("error in (no error)"=w393, "Generic Controller in"=w392) -> ("error out"=w391:errorcluster)  [unwired: 8 in, 1 out]
        }
        n184 = call "Ready Status.vi"("error in (no error)"=w384) -> ("error out"=w390:errorcluster)  [unwired: 2 in]
      }
      frame "Stop Hardware Run" {
        n185 = Unbundle By Name(w401) -> ("Hardware.Process Cache"=w400:refnum<class "Controller Array.lvclass">)
        n186 = call "Update Status.vi"("error in (no error)"=w398, "Status Bar Text"="Stopping hardware run.") -> ("error out"=w395:errorcluster)  [unwired: 9 in]
        n187 = call "Read Array.vi"("error in (no error)"=w395, "Controller Array in"=w400) -> ("error out"=w397:errorcluster, "Array"=w399:refnum<class "Generic Plugin.lvclass">[])  [unwired: 7 in, 1 out]
        n188 = for {
          tunnel: w399 -> [w404] mode=indexing
          shift-right: [w403] -> w396
          shift-left: w397 -> [w405]
          n189 = call "Send Stop Message.vi"("error in (no error)"=w405, "Generic Controller in"=w404) -> ("error out"=w403:errorcluster)  [unwired: 8 in, 1 out]
        }
        n190 = call "Ready Status.vi"("error in (no error)"=w396) -> ("error out"=w402:errorcluster)  [unwired: 2 in]
      }
      frame "Load Hardware" {
        w414 = "Select Hardware" ("Window Title")
        # "Load a selected process."
        n191 = Unbundle By Name(w420) -> ("Log Directory"=w416:path, "Hardware.Process Cache"=w417:refnum<class "Controller Array.lvclass">, "Hardware.Plugins"=w415:T4[])
        n192 = call "Update Status.vi"("error in (no error)"=w422, "Status Bar Text"="Loading Hardware...") -> ("error out"=w419:errorcluster)  [unwired: 9 in]
        n193 = call "Load Plugin Dialog.vi"("Plugin Selection Ring Text"=w414, "Window Title"=w414, "error in (no error)"=w419, "Plugin List"=w415) -> ("error out"=w411:errorcluster, "cancelled"=w413:bool, "Instance Name"=w409:string, "Plugin Selected"=w412:T4)  [unwired: 4 in]
        n194 = case shown="False" w413 {
          tunnel: w420 -> [w439 w450]
          tunnel: [w438 w450] -> w407
          tunnel: w417 -> [w437 _]
          tunnel: [w436 w449] -> w410
          tunnel: w411 -> [w430 w449]
          tunnel: w416 -> [w427 _]
          tunnel: w412 -> [w433 _]
          tunnel: w409 -> [w426 _]
          frame False {
            n195 = Unbundle By Name(w433) -> ("Controller Type"=w429:T5, "Control Panel Path"=w428:path)
            n196 = call "Initialize Plugin.vi"("Instance Name (blank for default)"=w426, "error in (no error)"=w430, "Log Directory"=w427, "Plugin Path in"=w428, "Plugin Type"=w429) -> ("error out"=w423:errorcluster, "Failed?"=w424:bool, "Generic Controller out"=w425:refnum<class "Generic Plugin.lvclass">)  [unwired: 4 in]
            n197 = case shown="False" w424 {
              tunnel: w437 -> [w444 w446]
              tunnel: [w443 w448] -> w432
              tunnel: [w442 w446] -> w431
              tunnel: w425 -> [w441 _]
              tunnel: w423 -> [w440 w445]
              frame False {
                n198 = call "Add Hardware.vi"("error in (no error)"=w440, "new plugin"=w441, "Plugin Array in"=w444) -> ("error out"=w443:errorcluster, "Plugin Array out"=w442:refnum<class "Controller Array.lvclass">)  [unwired: 7 in]
              }
              frame True {
                # "Clear \"VI already\nclosed\" error that\nsometimes occurs\non abort"
                n199 = call <vilib>:"Clear Errors.vi"("error in (no error)"=w445, "specific error code to clear (0: all)"=1026) -> ("error out"=w448:errorcluster)  [unwired: 4 in, 1 out]
              }
            }
            n200 = Bundle By Name(cluster=w439, "Hardware.Process Cache"=w431) -> (w438:T2)
            n201 = control-ref of="This VI"() -> (w435:refnum<vi>)
            n202 = call "Set Unsaved Changes in Title.vi"("VI in"=w435, "error in (no error)"=w432, "Unsaved changes? (F)"=TRUE) -> ("error out"=w436:errorcluster)  [unwired: 8 in]
          }
          frame True {
          }
        }
        n203 = Unbundle By Name(w407) -> ("Hardware.Process Cache"=w408:refnum<class "Controller Array.lvclass">)
        n204 = call "Array Size.vi"("Controller Array in"=w408) -> ("size(s)"=→"# of controllers cached":i32)  [unwired: 1 in, 2 out]
        n205 = call "Ready Status.vi"("error in (no error)"=w410) -> ("error out"=w418:errorcluster)  [unwired: 2 in]
      }
      frame "Load Analyzer" {
        w452 = "Select Analyzer"
        # "Keep the queue reference in memory until the process can\nstart receiving commands"
        # "Stop the current analyzer"
        n206 = Unbundle By Name(w467) -> ("Log Directory"=w456:path, "Analyzers.Process Cache"=w460:refnum<class "Controller Array.lvclass">, "Analyzers.Plugins"=w466:T4[])
        n207 = call "Update Status.vi"("error in (no error)"=w464, "Status Bar Text"="Loading Analyzer...") -> ("error out"=w463:errorcluster)  [unwired: 9 in]
        n208 = call "Load Plugin Dialog.vi"("Plugin Selection Ring Text"=w452, "Window Title"=w452, "error in (no error)"=w463, "Plugin List"=w466) -> ("error out"=w455:errorcluster, "cancelled"=w454:bool, "Instance Name"=w451:string, "Plugin Selected"=w453:T4)  [unwired: 4 in]
        n209 = case shown="False" w454 {
          tunnel: [w484 w494] -> w459
          tunnel: w467 -> [w483 w494]
          tunnel: w455 -> [w475 w495]
          tunnel: w460 -> [w482 _]
          tunnel: [w479 w495] -> w462
          tunnel: w456 -> [w471 _]
          tunnel: w453 -> [w476 _]
          tunnel: w451 -> [w470 _]
          frame False {
            n210 = Unbundle By Name(w476) -> ("Controller Type"=w472:T5, "Control Panel Path"=w473:path)
            n211 = call "Initialize Plugin.vi"("Instance Name (blank for default)"=w470, "error in (no error)"=w475, "Log Directory"=w471, "Plugin Path in"=w473, "Plugin Type"=w472) -> ("error out"=w474:errorcluster, "Failed?"=w468:bool, "Generic Controller out"=w469:refnum<class "Generic Plugin.lvclass">)  [unwired: 4 in]
            n212 = case shown="False" w468 {
              tunnel: w482 -> [w489 w490]
              tunnel: [w488 w490] -> w481
              tunnel: [w487 w491] -> w480
              tunnel: w474 -> [w486 w492]
              tunnel: w469 -> [w485 _]
              frame False {
                n213 = call "Add Analyzer.vi"("error in (no error)"=w486, "new plugin"=w485, "Plugin Array in"=w489) -> ("error out"=w487:errorcluster, "Plugin Array out"=w488:refnum<class "Controller Array.lvclass">)  [unwired: 7 in]
              }
              frame True {
                # "Clear \"VI already\nclosed\" error that\nsometimes occurs\non abort"
                n214 = call <vilib>:"Clear Errors.vi"("error in (no error)"=w492, "specific error code to clear (0: all)"=1026) -> ("error out"=w491:errorcluster)  [unwired: 4 in, 1 out]
              }
            }
            n215 = Bundle By Name(cluster=w483, "Analyzers.Process Cache"=w481) -> (w484:T2)
            n216 = control-ref of="This VI"() -> (w478:refnum<vi>)
            n217 = call "Set Unsaved Changes in Title.vi"("VI in"=w478, "error in (no error)"=w480, "Unsaved changes? (F)"=TRUE) -> ("error out"=w479:errorcluster)  [unwired: 8 in]
          }
          frame True {
          }
        }
        n218 = Unbundle By Name(w459) -> ("Analyzers.Process Cache"=w458:refnum<class "Controller Array.lvclass">)
        n219 = call "Array Size.vi"("Controller Array in"=w458) -> ("size(s)"=→"# of analyzers cached":i32)  [unwired: 1 in, 2 out]
        n220 = call "Ready Status.vi"("error in (no error)"=w462) -> ("error out"=w461:errorcluster)  [unwired: 2 in]
      }
      frame "Load Optimizer" {
        # "Right now we can only load one optimizer at a time, so check if one is already loaded\nin the process cache. If there is one, do not try to load another."
        # "Load a selected process."
        n221 = Unbundle By Name(w509) -> ("Log Directory"=w496:path, "Optimizers.Process Cache"=w500:refnum<class "Controller Array.lvclass">, "Optimizers.Plugins"=w508:T4[])
        n222 = call "Update Status.vi"("error in (no error)"=w506, "Status Bar Text"="Loading Optimizer...") -> ("error out"=w505:errorcluster)  [unwired: 9 in]
        n223 = call "Array Size.vi"("Controller Array in"=w500) -> ("size(s)"=w502:i32)  [unwired: 1 in, 2 out]
        n224 = Less Or Equal To 0?(x=w502) -> (x <= 0?=w501:bool)
        n225 = case shown="True" w501 {
          tunnel: [w511 w523] -> w499
          tunnel: w509 -> [w511 w522]
          tunnel: w508 -> [_ w516]
          tunnel: w505 -> [w510 w521]
          tunnel: w500 -> [_ w519]
          tunnel: [w510 w518] -> w504
          tunnel: w496 -> [_ w517]
          frame False {
          }
          frame True {
            w513 = "Select Optimizer"
            n226 = call "Load Plugin Dialog.vi"("Plugin Selection Ring Text"=w513, "Window Title"=w513, "error in (no error)"=w521, "Plugin List"=w516) -> ("error out"=w520:errorcluster, "cancelled"=w515:bool, "Instance Name"=w512:string, "Plugin Selected"=w514:T4)  [unwired: 4 in]
            n227 = case shown="False" w515 {
              tunnel: [w540 w551] -> w523
              tunnel: w522 -> [w539 w551]
              tunnel: w520 -> [w531 w552]
              tunnel: w519 -> [w538 _]
              tunnel: [w534 w552] -> w518
              tunnel: w517 -> [w527 _]
              tunnel: w514 -> [w532 _]
              tunnel: w512 -> [w526 _]
              frame False {
                n228 = Unbundle By Name(w532) -> ("Controller Type"=w529:T5, "Control Panel Path"=w528:path)
                n229 = call "Initialize Plugin.vi"("Instance Name (blank for default)"=w526, "error in (no error)"=w531, "Log Directory"=w527, "Plugin Path in"=w528, "Plugin Type"=w529) -> ("error out"=w530:errorcluster, "Failed?"=w524:bool, "Generic Controller out"=w525:refnum<class "Generic Plugin.lvclass">)  [unwired: 4 in]
                n230 = case shown="False" w524 {
                  tunnel: w538 -> [w546 w549]
                  tunnel: [w545 w549] -> w537
                  tunnel: [w543 w547] -> w535
                  tunnel: w530 -> [w542 w548]
                  tunnel: w525 -> [w541 _]
                  frame False {
                    n231 = control-ref of="Optimizer Control"() -> (w544:refnum<vi>)
                    n232 = call "Add Optimizer.vi"("Optimizer Control"=w544, "error in (no error)"=w542, "new plugin"=w541, "Plugin Array in"=w546) -> ("error out"=w543:errorcluster, "Plugin Array out"=w545:refnum<class "Controller Array.lvclass">)  [unwired: 6 in]
                  }
                  frame True {
                    # "Clear \"VI already\nclosed\" error that\nsometimes occurs\non abort"
                    n233 = call <vilib>:"Clear Errors.vi"("error in (no error)"=w548, "specific error code to clear (0: all)"=1026) -> ("error out"=w547:errorcluster)  [unwired: 4 in, 1 out]
                  }
                }
                n234 = Bundle By Name(cluster=w539, "Optimizers.Process Cache"=w537) -> (w540:T2)
                n235 = control-ref of="This VI"() -> (w536:refnum<vi>)
                n236 = call "Set Unsaved Changes in Title.vi"("VI in"=w536, "error in (no error)"=w535, "Unsaved changes? (F)"=TRUE) -> ("error out"=w534:errorcluster)  [unwired: 8 in]
              }
              frame True {
              }
            }
          }
        }
        n237 = Unbundle By Name(w499) -> ("Optimizers.Process Cache"=w498:refnum<class "Controller Array.lvclass">)
        n238 = call "Array Size.vi"("Controller Array in"=w498) -> ("size(s)"=→"# of optimizers cached":i32)  [unwired: 1 in, 2 out]
        n239 = call "Ready Status.vi"("error in (no error)"=w504) -> ("error out"=w503:errorcluster)  [unwired: 2 in]
      }
      frame "Stop Hardware" {
        w562 = "Closing hardware" ("Status Bar Text")
        # "Stop the selected process"
        n240 = Variant To Data(error in=w566, type=w562, Variant=w563) -> (data=w561:string, error out=w565:errorcluster)
        n241 = call "Update Status.vi"("Status Bar Text"=w562) -> ("error out"=w564:errorcluster)  [unwired: 10 in]
        n242 = Merge Errors(w564, w565) -> (w560:errorcluster)
        n243 = Unbundle By Name(w554) -> ("Hardware.Process Cache"=w557:refnum<class "Controller Array.lvclass">)
        n244 = call "Search Array.vi"("error in (no error)"=w560, "Search Value"=w561, "Controller Array in"=w557) -> ("error out"=w555:errorcluster, "Controller found"=w556:refnum<class "Generic Plugin.lvclass">, "Index of found"=w553:i32)  [unwired: 1 in, 1 out]
        n245 = case shown="Default" w553 {
          selector: w553 -> [_ w572]
          tunnel: w561 -> [_ w590]
          tunnel: [w568 w588] -> w559
          tunnel: [w569 w585] -> w558
          tunnel: w556 -> [_ w573]
          tunnel: w555 -> [w568 w582]
          tunnel: w554 -> [w569 w574]
          frame -1 {
            # "Do nothing if the plugin was not found"
          }
          frame Default {
            # "Check if it is the last element.\nIf so, the index may remain the\nsame. This also handles when\nthe last hardware is removed, as\nthe \"None\" option (index 0) will be\nselected.\n\nIf it is not the last element in the \nhardware list, then the hardware \nplugin after it is selected."
            # "Stop the hardware before trying\nto shut down the controller"
            n246 = call "Send Stop Message.vi"("error in (no error)"=w582, "Generic Controller in"=w573) -> ("error out"=w581:errorcluster)  [unwired: 8 in, 1 out]
            n247 = call "Stop Process VI.vi"("error in (no error)"=w581, "Blocking (T)"=TRUE, "Process Name"=w590, "Data in"=w574) -> ("error out"=w580:errorcluster, "Data out"=w585:T2)  [unwired: 6 in]
            n248 = Unbundle By Name(w585) -> ("Hardware.Process Cache"=w577:refnum<class "Controller Array.lvclass">)
            n249 = call "Hardware List Updated.vi"("error in (no error)"=w580) -> ("error out"=w578:errorcluster)  [unwired: 10 in]
            n250 = Unbundle By Name(w585) -> ("Message History"=w584:string[][])
            n251 = call "Array Size.vi"("Controller Array in"=w577, "error in (no error)"=w578) -> ("size(s)"=w570:i32, "error out"=w575:errorcluster)  [unwired: 1 out]
            n252 = property on="List of Running Plugins" class="MCListbox (strict)"("ItemNames"=w584) -> ()  [unwired: 2 in, 2 out]
            n253 = Equal?(x=w572, y=w570) -> (x = y?=w576:bool)
            n254 = local write "# of controllers cached"(w570) -> ()
            n255 = Increment(x=w572) -> (x+1=w571:i32)
            n256 = Select(t=w572, s=w576, f=w571) -> (s? t:f=w579:i32)
            n257 = call "New Hardware Selected.vi"("error in (no error)"=w575, "Hardware Index"=w579) -> ("error out"=w586:errorcluster)  [unwired: 9 in]
            n258 = control-ref of="This VI"() -> (w589:refnum<vi>)
            n259 = call "Set Unsaved Changes in Title.vi"("VI in"=w589, "error in (no error)"=w586, "Unsaved changes? (F)"=TRUE) -> ("error out"=w588:errorcluster)  [unwired: 8 in]
          }
        }
        n260 = call "Ready Status.vi"("error in (no error)"=w559) -> ("error out"=w567:errorcluster)  [unwired: 2 in]
      }
      frame "Stop Analyzer" {
        w603 = "Closing analyzer" ("Status Bar Text")
        # "Stop the analyzer and remove it from the subpanel."
        n261 = Variant To Data(error in=w602, type=w603, Variant=w600) -> (data=w591:string, error out=w605:errorcluster)
        n262 = call "Update Status.vi"("Status Bar Text"=w603) -> ("error out"=w604:errorcluster)  [unwired: 10 in]
        n263 = Merge Errors(w604, w605) -> (w596:errorcluster)
        n264 = Unbundle By Name(w598) -> ("Analyzers.Process Cache"=w595:refnum<class "Controller Array.lvclass">)
        n265 = call "Search Array.vi"("error in (no error)"=w596, "Search Value"=w591, "Controller Array in"=w595) -> ("error out"=w594:errorcluster, "Controller found"=w593:refnum<class "Generic Plugin.lvclass">, "Index of found"=w592:i32)  [unwired: 1 in, 1 out]
        n266 = case shown="Default" w592 {
          selector: w592 -> [_ w611]
          tunnel: [w607 w625] -> w599
          tunnel: w598 -> [w607 w624]
          tunnel: [w606 w620] -> w597
          tunnel: w594 -> [w606 w619]
          tunnel: w593 -> [_ _]
          tunnel: w591 -> [_ w618]
          frame -1 {
            # "Do nothing if plugin was not found"
          }
          frame Default {
            # "Check if it is the last element.\nIf so, the index may remain the\nsame. This also handles when\nthe last hardware is removed, as\nthe \"None\" option (index 0) will be\nselected.\n\nIf it is not the last element in the \nanalyzer list, then the analyzer \nplugin after it is selected."
            n267 = call "Stop Analyzer VI.vi"("error in (no error)"=w619, "Blocking (T)"=TRUE, "Process Name"=w618, "Data in"=w624) -> ("error out"=w617:errorcluster, "Data out"=w625:T2)  [unwired: 6 in]
            n268 = Unbundle By Name(w625) -> ("Message History"=w616:string[][], "Analyzers.Process Cache"=w623:refnum<class "Controller Array.lvclass">)
            n269 = call "Analyzer List Updated.vi"("error in (no error)"=w617) -> ("error out"=w615:errorcluster)  [unwired: 10 in]
            n270 = property on="List of Running Plugins" class="MCListbox (strict)"("ItemNames"=w616) -> ()  [unwired: 2 in, 2 out]
            n271 = call "Array Size.vi"("Controller Array in"=w623, "error in (no error)"=w615) -> ("size(s)"=w612:i32, "error out"=w610:errorcluster)  [unwired: 1 out]
            n272 = local write "# of analyzers cached"(w612) -> ()
            n273 = Equal?(x=w611, y=w612) -> (x = y?=w614:bool)
            n274 = Increment(x=w611) -> (x+1=w613:i32)
            n275 = Select(t=w611, s=w614, f=w613) -> (s? t:f=w609:i32)
            n276 = call "New Analyzer Selected.vi"("error in (no error)"=w610, "Analyzer Index"=w609) -> ("error out"=w608:errorcluster)  [unwired: 9 in]
            n277 = control-ref of="This VI"() -> (w622:refnum<vi>)
            n278 = call "Set Unsaved Changes in Title.vi"("VI in"=w622, "error in (no error)"=w608, "Unsaved changes? (F)"=TRUE) -> ("error out"=w620:errorcluster)  [unwired: 8 in]
          }
        }
        n279 = call "Ready Status.vi"("error in (no error)"=w597) -> ("error out"=w601:errorcluster)  [unwired: 2 in]
      }
      frame "Stop Optimizer" {
        w648 = "Closing optimizer" ("Status Bar Text")
        # "Remove VI from subpanel"
        # "Stop the current optimizer"
        n280 = Variant To Data(error in=w647, type=w648, Variant=w645) -> (error out=w650:errorcluster)  [unwired: 1 out]
        n281 = call "Update Status.vi"("Status Bar Text"=w648) -> ("error out"=w649:errorcluster)  [unwired: 10 in]
        n282 = Merge Errors(w649, w650) -> (w637:errorcluster)
        n283 = Unbundle By Name(w640) -> ("Optimizers.Process Cache"=w639:refnum<class "Controller Array.lvclass">)
        n284 = call "Index Array.vi"("error in (no error)"=w637, "index"=0, "Controller Array in"=w639) -> ("error out"=w635:errorcluster, "element"=w636:refnum<class "Generic Plugin.lvclass">)  [unwired: 1 out]
        n285 = call "Read Name.vi"("controller in"=w636, "error in (no error)"=w635) -> ("Name"=w633:string, "error out"=w634:errorcluster)  [unwired: 1 out]
        n286 = call "Stop Optimizer VI.vi"("error in (no error)"=w634, "Blocking (T)"=TRUE, "Process Name"=w633, "Data in"=w640) -> ("error out"=w644:errorcluster, "Data out"=w641:T2)  [unwired: 6 in]
        n287 = Unbundle By Name(w641) -> ("Optimizers.Process Cache"=w632:refnum<class "Controller Array.lvclass">, "Message History"=w642:string[][])
        n288 = call "Array Size.vi"("Controller Array in"=w632) -> ("size(s)"=w631:i32)  [unwired: 1 in, 2 out]
        n289 = property on="List of Running Plugins" class="MCListbox (strict)"("ItemNames"=w642) -> ()  [unwired: 2 in, 2 out]
        n290 = local write "# of optimizers cached"(w631) -> ()
        n291 = invoke on="Optimizer Control" class="SubPnl" method="Remove VI"(error in=w644) -> (error out=w629:errorcluster)  [unwired: 2 in, 2 out]
        n292 = control-ref of="This VI"() -> (w630:refnum<vi>)
        n293 = call "Set Unsaved Changes in Title.vi"("VI in"=w630, "error in (no error)"=w629, "Unsaved changes? (F)"=TRUE) -> ("error out"=w628:errorcluster)  [unwired: 8 in]
        n294 = call "Ready Status.vi"("error in (no error)"=w628) -> ("error out"=w646:errorcluster)  [unwired: 2 in]
      }
      frame "New Parameters" {
        # "If this is the first time receiving parameters from the reactor control plugin, populate the keys of the Parameter to Hardware Map with the names of the parameters."
        # "Register new parameters from a reactor control plugin with Rxn Rover, preparing them to be sent to hardware plugins."
        n295 = Unbundle By Name(w666) -> ("Optimizers.First parameteres?"=w665:bool, "Parameter to Hardware Map"=w663:refnum<class "Parameter to Hardware Map.lvclass">, "Hardware.Process Cache"=w661:refnum<class "Controller Array.lvclass">)
        n296 = Variant To Data(error in=w664, type=T8 {"Time Stamp"=timestamp(0 s since 1904-01-01), "Names"=[], "Values"=[]} ("New Parameters"), Variant=w659) -> (data=w657:T8, error out=w660:errorcluster)
        n297 = case shown="True" w665 {
          selector: w665 -> [w677 _]
          tunnel: w660 -> [w679 w689]
          tunnel: [w679 w680] -> w655
          tunnel: w663 -> [w678 w691]
          tunnel: w657 -> [_ w690]
          tunnel: w661 -> [_ w687]
          tunnel: [w678 w686] -> w662
          tunnel: [w677 FALSE] -> w658
          frame False {
          }
          frame True {
            n298 = Unbundle By Name(w690) -> ("Names"=w685:string[])
            n299 = for {
              tunnel: w685 -> [w692] mode=indexing
              shift-right: [w694] -> w681
              shift-left: w689 -> [w695]
              shift-right: [w693] -> w688
              shift-left: w691 -> [w696]
              n300 = call "Insert (key-value).vi"("error in (no error)"=w695, "Key"=w692, "Parameter to Hardware Map in"=w696) -> ("error out"=w694:errorcluster, "Parameter to Hardware Map out"=w693:refnum<class "Parameter to Hardware Map.lvclass">)  [unwired: 7 in]
            }
            n301 = call "Assign Parameters to Hardware Dialog.vi"("Hardware Object List"=w687, "Parameter to Hardware Map in"=w688) -> ("Parameter to Hardware Map out"=w686:refnum<class "Parameter to Hardware Map.lvclass">)  [unwired: 9 in]
            n302 = control-ref of="This VI"() -> (w683:refnum<vi>)
            n303 = call "Set Unsaved Changes in Title.vi"("VI in"=w683, "error in (no error)"=w681, "Unsaved changes? (F)"=TRUE) -> ("error out"=w680:errorcluster)  [unwired: 8 in]
          }
        }
        n304 = Bundle By Name(cluster=w666, "Optimizers.First parameteres?"=w658, "Parameter to Hardware Map"=w662, "Optimizers.New Parameters"=w657) -> (w653:T2)
        n305 = Unbundle By Name(w653) -> ("Auto Pass Parameters"=w652:bool)
        n306 = case shown="False" w652 {
          tunnel: w656 -> [_ w674]
          tunnel: w655 -> [w670 w676]
          tunnel: [w670 w675] -> w654
          frame False {
            w668 = FALSE  # Un-press buttons
            w669 = T15."Enabled"  # Enable Buttons
            # "Enable the Accept and Reject Parameter buttons on the UI."
            n307 = property on="Accept Suggestions" class="Bool (strict)"("DisabledEnum"=w669, "Value"=w668) -> ()  [unwired: 2 in, 2 out]
            n308 = property on="Reject Suggestions" class="Bool (strict)"("DisabledEnum"=w669, "Value"=w668) -> ()  [unwired: 2 in, 2 out]
          }
          frame True {
            w672 = FALSE  # Un-press buttons
            w671 = T15."Disabled and Grayed Out"  # Disable Buttons
            # "Automatically send the parameters to the hardware if the user toggled it on"
            n309 = call-poly "Enqueue Message.vi"("error in (no error)"=w676, "Message"="Send Parameters", "Message Queue"=w674) -> ("error out"=w675:errorcluster)  [unwired: 7 in, 1 out]
            n310 = property on="Accept Suggestions" class="Bool (strict)"("DisabledEnum"=w671, "Value"=w672) -> ()  [unwired: 2 in, 2 out]
            n311 = property on="Reject Suggestions" class="Bool (strict)"("DisabledEnum"=w671, "Value"=w672) -> ()  [unwired: 2 in, 2 out]
          }
        }
        n312 = call "Ready Status.vi"("error in (no error)"=w654) -> ("error out"=w667:errorcluster)  [unwired: 2 in]
      }
      frame "Send Parameters" {
        # "Parameter to Hardware Map is set when the user presses the \"Reassign Parameters\" button or after being prompted the first time Rxn Rover receives parameters."
        # "Send the optimizer's suggested parameter values to the assigned hardware."
        n313 = Unbundle By Name(w699) -> ("Optimizers.First parameteres?"=w698:bool)
        n314 = Unbundle By Name(w699) -> ("Parameter to Hardware Map"=w705:refnum<class "Parameter to Hardware Map.lvclass">, "Optimizers.New Parameters"=w702:T8)
        n315 = call "Update Status.vi"("error in (no error)"=w707, "Status Bar Text"="Broadcasting reaction parameters.") -> ("error out"=w704:errorcluster)  [unwired: 9 in]
        n316 = Unbundle By Name(w702) -> ("Names"=w700:string[], "Values"=w701:variant[])
        n317 = case shown="True" w698 {
          frame False {
            w708 = T15."Disabled and Grayed Out" ("Disabled")
            n318 = property on="Accept Suggestions" class="Bool (strict)"("DisabledEnum"=w708, "Value"=TRUE ("Accept Suggestions")) -> ()  [unwired: 2 in, 2 out]
            n319 = property on="Reject Suggestions" class="Bool (strict)"("DisabledEnum"=w708) -> ()  [unwired: 2 in, 2 out]
          }
          frame True {
            n320 = property on="Accept Suggestions" class="Bool (strict)"("Value"=FALSE ("Accept Suggestions")) -> ()  [unwired: 2 in, 2 out]
          }
        }
        n321 = for {
          tunnel: w705 -> [w718]
          shift-right: [w713] -> w703
          shift-left: w704 -> [w715]
          tunnel: w701 -> [w712] mode=indexing
          tunnel: w700 -> [w711] mode=indexing
          # "For each parameter..."
          n322 = call "Find (single).vi"("error in (no error)"=w715, "Key"=w711, "Parameter to Hardware Map in"=w718) -> ("error out"=w714:errorcluster, "Key-Value Pair"=w717:T16)  [unwired: 5 in, 2 out]
          n323 = Unbundle By Name(w717) -> ("values"=w716:refnum<class "Generic Plugin.lvclass">[])
          n324 = for {
            tunnel: w716 -> [w722] mode=indexing
            shift-right: [w719] -> w713
            shift-left: w714 -> [w721]
            tunnel: w712 -> [w720]
            # "...send the value to each assigned plugin"
            n325 = call "Send New Parameter.vi"("error in (no error)"=w721, "New parameter"=w720, "controller in"=w722) -> ("error out"=w719:errorcluster)  [unwired: 7 in, 1 out]
          }
        }
        n326 = call "Ready Status.vi"("error in (no error)"=w703) -> ("error out"=w697:errorcluster)  [unwired: 2 in]
      }
      frame "Reject Parameters" {
        # "Reject the optimizer's suggested values"
        n327 = Unbundle By Name(w727) -> ("Optimizers.First parameteres?"=w726:bool)
        n328 = call "Update Status.vi"("error in (no error)"=w729, "Status Bar Text"="Rejecting suggestions; Requesting new ones.") -> ("error out"=w725:errorcluster)  [unwired: 9 in]
        n329 = case shown="False" w726 {
          tunnel: w725 -> [w734 w737]
          tunnel: w723 -> [w731 _]
          tunnel: [w730 w737] -> w724
          frame False {
            w735 = T15."Disabled and Grayed Out" ("Disabled")
            # "Punish optimizer for going\nout of range"
            n330 = call-poly "Enqueue Message.vi"("error in (no error)"=w734, "Message Data"=-1.0, "Message"="Submit Goal", "Message Queue"=w731) -> ("error out"=w730:errorcluster)  [unwired: 6 in, 1 out]
            n331 = property on="Accept Suggestions" class="Bool (strict)"("DisabledEnum"=w735) -> ()  [unwired: 2 in, 2 out]
            n332 = property on="Reject Suggestions" class="Bool (strict)"("DisabledEnum"=w735, "Value"=TRUE ("Reject Suggestions")) -> ()  [unwired: 2 in, 2 out]
          }
          frame True {
            n333 = property on="Reject Suggestions" class="Bool (strict)"("Value"=FALSE ("Reject Suggestions")) -> ()  [unwired: 2 in, 2 out]
          }
        }
      }
      frame "Reassign Parameters" {
        # "Reassign parameters to instruments in the Parameter to Hardware Map"
        n334 = Unbundle By Name(w756) -> ("Hardware.Process Cache"=w753:refnum<class "Controller Array.lvclass">, "Optimizers.New Parameters"=w752:T8)
        n335 = call "Update Status.vi"("error in (no error)"=w755, "Status Bar Text"="Reassigning parameters") -> ("error out"=w750:errorcluster)  [unwired: 9 in]
        n336 = Unbundle By Name(w752) -> ("Names"=w742:string[])
        n337 = for {
          tunnel: w742 -> [w758] mode=indexing
          shift-right: [w760] -> w739
          shift-left: w750 -> [w761]
          shift-right: [w759] -> w743
          shift-left: refnum<class "Parameter to Hardware Map.lvclass"> refnum ("Parameter to Hardware Map") -> [w762]
          n338 = call "Insert (key-value).vi"("error in (no error)"=w761, "Key"=w758, "Parameter to Hardware Map in"=w762) -> ("error out"=w760:errorcluster, "Parameter to Hardware Map out"=w759:refnum<class "Parameter to Hardware Map.lvclass">)  [unwired: 7 in]
        }
        n339 = call "Assign Parameters to Hardware Dialog.vi"("Hardware Object List"=w753, "Parameter to Hardware Map in"=w743) -> ("Parameter to Hardware Map out"=w754:refnum<class "Parameter to Hardware Map.lvclass">)  [unwired: 9 in]
        n340 = control-ref of="This VI"() -> (w741:refnum<vi>)
        n341 = call "Set Unsaved Changes in Title.vi"("VI in"=w741, "error in (no error)"=w739, "Unsaved changes? (F)"=TRUE) -> ("error out"=w748:errorcluster)  [unwired: 8 in]
        n342 = Bundle By Name(cluster=w756, "Parameter to Hardware Map"=w754) -> (w745:T2)
        n343 = Unbundle By Name(w745) -> ("Auto Pass Parameters"=w744:bool)
        n344 = case shown="True" w744 {
          tunnel: w746 -> [_ w768]
          tunnel: w748 -> [w766 w770]
          tunnel: [w766 w769] -> w747
          frame False {
            w765 = T15."Enabled" ("Disabled")
            n345 = property on="Accept Suggestions" class="Bool (strict)"("DisabledEnum"=w765, "Value"=FALSE ("Accept Suggestions")) -> ()  [unwired: 2 in, 2 out]
            n346 = property on="Reject Suggestions" class="Bool (strict)"("DisabledEnum"=w765, "Value"=FALSE ("Reject Suggestions")) -> ()  [unwired: 2 in, 2 out]
          }
          frame True {
            n347 = call-poly "Enqueue Message.vi"("error in (no error)"=w770, "Message"="Send Parameters", "Message Queue"=w768) -> ("error out"=w769:errorcluster)  [unwired: 7 in, 1 out]
          }
        }
        n348 = call "Ready Status.vi"("error in (no error)"=w747) -> ("error out"=w757:errorcluster)  [unwired: 2 in]
      }
      frame "Toggle Auto Param Passing" {
        # "Toggles whether parameters are passed automatically or not."
        n349 = Variant To Data(error in=w776, type=FALSE, Variant=w773) -> (data=w771:bool, error out=w774:errorcluster)
        n350 = Bundle By Name(cluster=w777, "Auto Pass Parameters"=w771) -> (w775:T2)
      }
      frame "Submit Goal" {
        # "Submit the goal value(s) to the optimizer(s)"
        n351 = Unbundle By Name(w782) -> ("Optimizers.Process Cache"=w781:refnum<class "Controller Array.lvclass">)
        n352 = call "Array Size.vi"("Controller Array in"=w781) -> ("size(s)"=w779:i32)  [unwired: 1 in, 2 out]
        n353 = Greater Than 0?(x=w779) -> (x > 0?=w780:bool)
        n354 = case shown="True" w780 {
          tunnel: w785 -> [w786 w802]
          tunnel: [w786 w800] -> w784
          tunnel: w783 -> [_ w798]
          tunnel: w781 -> [_ w794]
          frame False {
          }
          frame True {
            w791 = refnum<class "Generic Optimizer.lvclass"> refnum  # Generic Optimizer.lvclass
            n355 = call "Update Status.vi"("error in (no error)"=w802, "Status Bar Text"="Submitting yield") -> ("error out"=w803:errorcluster)  [unwired: 9 in]
            n356 = call "Search Array.vi"("Searchable Property (Name)"=Searchable_Properties."Controller Type", "Search Value"=Controller_Type."Generic Optimizer" ("Controller Type"), "Controller Array in"=w794) -> ("error out"=w789:errorcluster, "Controller found"=w792:refnum<class "Generic Plugin.lvclass">)  [unwired: 1 in, 2 out]
            n357 = Variant To Data(error in=w803, type=0.0, Variant=w798) -> (data=w796:dbl, error out=w799:errorcluster)
            n358 = To More Specific Class(target class=w791, reference=w792, error in=w789) -> (specific class reference=w790:refnum<class "Generic Optimizer.lvclass">, error out=w787:errorcluster)
            n359 = Merge Errors(w787, w799) -> (w788:errorcluster)
            n360 = call-dynamic "Submit Goal.vi"("error in (no error)"=w788, "Goal"=w796, "Generic Optimizer in"=w790) -> ("error out"=w800:errorcluster)  [unwired: 7 in, 1 out]
          }
        }
        n361 = call "Ready Status.vi"("error in (no error)"=w784) -> ("error out"=w778:errorcluster)  [unwired: 2 in]
      }
    }
    n362 = call "Error Handler - Main VI State Machine.vi"("error in (no error)"=w45, "Message Queue"=w43) -> ("dup error in"=w44:errorcluster)  [unwired: 8 in, 1 out]
  }
  n363 = while {
    tunnel: w36 -> [w807]
    tunnel: w35 -> [w805]
    tunnel: [w804] -> w32
    stop <- w806 stop-if-true
    n364 = event shown="[31] \"Reorder Analyzers\": Value Change" {
      selector: w805 -> [_ _ _ _ _ _ _ _ _ _ _ _ _ _ _ _ _ _ _ _ _ _ _ _ _ _ _ _ _ _ _ _ _]
      dyn-events: [_ _ _ _ _ _ _ _ _ _ _ _ _ _ _ _ _ _ _ _ _ _ _ _ _ _ _ _ _ _ _ _ _] -> w804
      timeout: _ -> [_ _ _ _ _ _ _ _ _ _ _ _ _ _ _ _ _ _ _ _ _ _ _ _ _ _ _ _ _ _ _ _ _]
      tunnel: w807 -> [w810 _ w812 w816 w823 _ _ _ w831 w842 w847 _ w856 w858 w862 w865 w867 w869 w871 w874 w877 w879 w881 _ w889 w892 w895 w900 _ w912 w914 w915 w919]
      tunnel: [_ _ _ _ _ w826 _ _ _ _ _ _ _ _ _ _ _ _ _ _ _ _ _ _ _ _ _ _ _ _ _ _ _] -> w806
      event "Exit": Value Change {
        # "Begin the exitting process"
        n365 = event-data() -> ()  [unwired: 1 in, 1 out]
        n366 = call-poly "Enqueue Message.vi"("Priority Message? (F)"=TRUE, "Message"="Exitting", "Message Queue"=w810) -> ()  [unwired: 7 in, 2 out]
      }
      event Timeout {
        # "Do nothing on timeout. If no timeout value is given, this should not even be invoked."
        n367 = event-data() -> ()  [unwired: 1 in, 1 out]
      }
      event Application Instance Close {
        n368 = event-data() -> ()  [unwired: 1 in, 1 out]
        n369 = call-poly "Enqueue Message.vi"("Priority Message? (F)"=TRUE, "Message"="Exitting", "Message Queue"=w812) -> ()  [unwired: 7 in, 2 out]
      }
      event Panel Close? {
        n370 = event-data() -> ()  [unwired: 1 in, 1 out]
        n371 = call-poly "Enqueue Message.vi"("Priority Message? (F)"=TRUE, "Message"="Exitting", "Message Queue"=w816) -> ()  [unwired: 7 in, 2 out]
        n372 = event-data("Discard?"=TRUE) -> ()  [unwired: 1 in, 1 out]
      }
      event Key Down {
        w822 = 115  # 's' key
        n373 = event-data() -> ("Char"=w821:i16, "Mods.Menu Key"=w818:bool)  [unwired: 1 in]
        n374 = Equal?(x=w822, y=w821) -> (x = y?=w819:bool)
        n375 = And(x=w819, y=w818) -> (x .and. y?=w820:bool)
        n376 = case shown="True" w820 {
          tunnel: w823 -> [_ w825]
          frame False {
          }
          frame True {
            n377 = call-poly "Enqueue Message.vi"("Message"="Save Experiment", "Message Queue"=w825) -> ()  [unwired: 8 in, 2 out]
          }
        }
      }
      event User Event {
        n378 = event-data() -> ("Stop"=w826:bool)  [unwired: 1 in]
      }
      event User Event {
        n379 = event-data() -> ("Status"=→"Status Bar Text":string)  [unwired: 1 in]
      }
      event User Event {
        n380 = event-data() -> ("VIs"=w829:refnum<class "Controller Array.lvclass">)  [unwired: 1 in]
        n381 = call "Array Size.vi"("Controller Array in"=w829) -> ("size(s)"=→"# of plugins cached":i32)  [unwired: 1 in, 2 out]
      }
      event User Event {
        n382 = event-data() -> ("Source"=w837:string, "Destination"=w836:string, "Time Stamp"=w835:timestamp, "Command"=w834:string, "Data"=w833:variant)  [unwired: 1 in]
        n383 = Bundle By Name(cluster=T3 {"Source"="", "Destination"="", "Time Stamp"=timestamp(0 s since 1904-01-01), "Command"="", "Data"=variant} ("Message"), "Source"=w837, "Destination"=w836, "Time Stamp"=w835, "Command"=w834, "Data"=w833) -> (w830:T3)
        n384 = call-poly "Enqueue Message.vi"("Message Data"=w830, "Message"="Cache Message", "Message Queue"=w831) -> ()  [unwired: 7 in, 2 out]
      }
      event User Event {
        # "Stop the selected controller"
        n385 = event-data() -> ("Type"=w839:enum16{"Hardware", "Optimizer", "Analyzer"}, "Name"=w840:string)  [unwired: 1 in]
        n386 = case shown="\"Hardware\", Default" w839 {
          tunnel: ["Stop Hardware" ("Message") "Stop Optimizer" ("Message") "Stop Analyzer" ("Message")] -> w841
          frame "Hardware", Default {
          }
          frame "Optimizer" {
          }
          frame "Analyzer" {
          }
        }
        n387 = call-poly "Enqueue Message.vi"("Message Data"=w840, "Message"=w841, "Message Queue"=w842) -> ()  [unwired: 7 in, 2 out]
      }
      event "Load Control Panel": Value Change {
        # "Send message to load controller"
        n388 = event-data() -> ()  [unwired: 1 in, 1 out]
        n389 = call-poly "Enqueue Message.vi"("Message"="Load Hardware", "Message Queue"=w847) -> ()  [unwired: 8 in, 2 out]
      }
      event "Stop Controller Btn": Value Change {
        # "Stop the selected controller"
        n390 = event-data() -> ()  [unwired: 1 in, 1 out]
        n391 = local read "Select a Plugin"() -> (w848:u16)
        n392 = case shown="Default" w848 {
          selector: w848 -> [_ w850]
          frame 0 {
            # "Do nothing if no plugin is selected"
          }
          frame Default {
            # "Fire a Process Stopped Event, providing\nthe name of the process to be stopped"
            n393 = property on="Select a Plugin" class="Ring (strict)"() -> ("Strings []"=w851:string[])  [unwired: 2 in, 2 out]
            n394 = Index Array(array=w851, index=w850) -> (element=w849:string)
            n395 = Bundle By Name(cluster=T17 {"Name"="", "Type"=enum."Hardware"} ("Process Cluster"), "Name"=w849, "Type"=enum16{"Hardware", "Optimizer"}."Hardware") -> (w852:T17)
            n396 = call "Process Stopped Event.vi"() -> ("Process Stopped"=w855:refnum<user-event>)  [unwired: 11 in]
            n397 = Generate User Event(user event=w855, event data cluster=w852) -> ()  [unwired: 2 in, 2 out]
          }
        }
      }
      event "Start Hardware Run Btn": Value Change {
        n398 = event-data() -> ()  [unwired: 1 in, 4 out]
        n399 = call-poly "Enqueue Message.vi"("Message"="Start Hardware Run", "Message Queue"=w856) -> ()  [unwired: 8 in, 2 out]
      }
      event "Stop Hardware Run Btn": Value Change {
        n400 = event-data() -> ()  [unwired: 1 in, 4 out]
        n401 = call-poly "Enqueue Message.vi"("Message"="Stop Hardware Run", "Message Queue"=w858) -> ()  [unwired: 8 in, 2 out]
      }
      event "Select a Plugin": Value Change {
        n402 = event-data() -> ("NewVal"=w861:u16)  [unwired: 1 in]
        n403 = call-poly "Enqueue Message.vi"("Message Data"=w861, "Message"="New Hardware Selected", "Message Queue"=w862) -> ()  [unwired: 7 in, 2 out]
      }
      event "View an Analyzer": Value Change {
        n404 = event-data() -> ("NewVal"=w864:u16)  [unwired: 1 in]
        n405 = call-poly "Enqueue Message.vi"("Message Data"=w864, "Message"="New Analyzer Selected", "Message Queue"=w865) -> ()  [unwired: 7 in, 2 out]
      }
      event User Event {
        n406 = event-data() -> ("Hardware Index"=w866:i32)  [unwired: 1 in]
        n407 = call-poly "Enqueue Message.vi"("Message Data"=w866, "Message"="New Hardware Selected", "Message Queue"=w867) -> ()  [unwired: 7 in, 2 out]
      }
      event User Event {
        n408 = event-data() -> ()  [unwired: 1 in, 1 out]
        n409 = call-poly "Enqueue Message.vi"("Message"="Refresh Hardware Selector", "Message Queue"=w869) -> ()  [unwired: 8 in, 2 out]
      }
      event User Event {
        n410 = event-data() -> ("Hardware Index"=w872:i32)  [unwired: 1 in]
        n411 = call-poly "Enqueue Message.vi"("Message Data"=w872, "Message"="New Analyzer Selected", "Message Queue"=w871) -> ()  [unwired: 7 in, 2 out]
      }
      event User Event {
        n412 = event-data() -> ()  [unwired: 1 in, 1 out]
        n413 = call-poly "Enqueue Message.vi"("Message"="Refresh Analyzer Selector", "Message Queue"=w874) -> ()  [unwired: 8 in, 2 out]
      }
      event "Accept Suggestions": Value Change {
        n414 = event-data() -> ()  [unwired: 1 in, 1 out]
        n415 = call-poly "Enqueue Message.vi"("Message"="Send Parameters", "Message Queue"=w877) -> ()  [unwired: 8 in, 2 out]
      }
      event "Reject Suggestions": Value Change {
        n416 = event-data() -> ()  [unwired: 1 in, 1 out]
        n417 = call-poly "Enqueue Message.vi"("Message"="Reject Parameters", "Message Queue"=w879) -> ()  [unwired: 8 in, 2 out]
      }
      event "Load Optimizer Btn": Value Change {
        n418 = event-data() -> ()  [unwired: 1 in, 1 out]
        n419 = call-poly "Enqueue Message.vi"("Message"="Load Optimizer", "Message Queue"=w881) -> ()  [unwired: 8 in, 2 out]
      }
      event "Stop Optimizer Btn": Value Change {
        # "Fire a Process Stopped Event, leaving\nthe process name blank so it is\ndetermined by the current process"
        n420 = event-data() -> ()  [unwired: 1 in, 1 out]
        n421 = Bundle By Name(cluster=T17 {"Name"="", "Type"=enum."Hardware"} ("Process Cluster"), "Name"="", "Type"=enum16{"Hardware", "Optimizer"}."Optimizer") -> (w885:T17)
        n422 = call "Process Stopped Event.vi"() -> ("Process Stopped"=w886:refnum<user-event>)  [unwired: 11 in]
        n423 = Generate User Event(user event=w886, event data cluster=w885) -> ()  [unwired: 2 in, 2 out]
      }
      event "Auto Param Passing": Value Change {
        n424 = event-data() -> ()  [unwired: 1 in, 1 out]
        n425 = call-poly "Enqueue Message.vi"("Message Data"="Auto Param Passing", "Message"="Toggle Auto Param Passing", "Message Queue"=w889) -> ()  [unwired: 7 in, 2 out]
      }
      event User Event {
        n426 = event-data() -> ("Goal"=w890:dbl)  [unwired: 1 in]
        n427 = call-poly "Enqueue Message.vi"("Message Data"=w890, "Message"="Submit Goal", "Message Queue"=w892) -> ()  [unwired: 7 in, 2 out]
      }
      event User Event {
        n428 = event-data() -> ("Time Stamp"=w898:timestamp, "Names"=w897:string[], "Values"=w896:variant[])  [unwired: 1 in]
        n429 = Bundle By Name(cluster=T8 {"Time Stamp"=timestamp(0 s since 1904-01-01), "Names"=[], "Values"=[]} ("New Parameters"), "Time Stamp"=w898, "Names"=w897, "Values"=w896) -> (w894:T8)
        n430 = call-poly "Enqueue Message.vi"("Message Data"=w894, "Message"="New Parameters", "Message Queue"=w895) -> ()  [unwired: 7 in, 2 out]
      }
      event "Load Analyzer Btn": Value Change {
        n431 = event-data() -> ()  [unwired: 1 in, 1 out]
        n432 = call-poly "Enqueue Message.vi"("Message"="Load Analyzer", "Message Queue"=w900) -> ()  [unwired: 8 in, 2 out]
      }
      event "Stop Analyzer Btn": Value Change {
        n433 = event-data() -> ()  [unwired: 1 in, 1 out]
        n434 = local read "View an Analyzer"() -> (w902:u16)
        n435 = case shown="Default" w902 {
          selector: w902 -> [_ w904]
          frame 0 {
          }
          frame Default {
            # "Fire a Process Stopped Event, leaving\nthe process name blank so it is\ndetermined by the current process"
            n436 = property on="View an Analyzer" class="Ring (strict)"() -> ("Strings []"=w905:string[])  [unwired: 2 in, 2 out]
            n437 = Index Array(array=w905, index=w904) -> (element=w903:string)
            n438 = Bundle By Name(cluster=T17 {"Name"="", "Type"=enum."Hardware"} ("Process Cluster"), "Name"=w903, "Type"=enum16{"Hardware", "Optimizer", "Analyzer"}."Analyzer") -> (w908:T17)
            n439 = call "Process Stopped Event.vi"() -> ("Process Stopped"=w909:refnum<user-event>)  [unwired: 11 in]
            n440 = Generate User Event(user event=w909, event data cluster=w908) -> ()  [unwired: 2 in, 2 out]
          }
        }
      }
      event User Event {
        # "Forward the new yield to the optimizer."
        n441 = event-data() -> ("New Yield"=w911:dbl)  [unwired: 1 in]
        n442 = call-poly "Enqueue Message.vi"("Message Data"=w911, "Message"="Submit Goal", "Message Queue"=w912) -> ()  [unwired: 7 in, 2 out]
      }
      event "Reassign Parameters": Value Change {
        # "Forward the new yield to the optimizer."
        n443 = event-data() -> ()  [unwired: 1 in, 1 out]
        n444 = call-poly "Enqueue Message.vi"("Message"="Reassign Parameters", "Message Queue"=w914) -> ()  [unwired: 8 in, 2 out]
      }
      event "Reorder Analyzers": Value Change {
        n445 = event-data() -> ()  [unwired: 1 in, 6 out]
        n446 = call-poly "Enqueue Message.vi"("Message"="Reorder Analyzers", "Message Queue"=w915) -> ()  [unwired: 8 in, 2 out]
      }
      event User Event {
        n447 = event-data() -> ("Path"=w918:path)  [unwired: 1 in]
        n448 = call-poly "Enqueue Message.vi"("Message Data"=w918, "Message"="New Log Path", "Message Queue"=w919) -> ()  [unwired: 7 in, 2 out]
      }
    }
  }
  n449 = disable-structure shown="Enabled" {
    frame Enabled {
    }
    frame Disabled {
    }
  }
  n450 = call "Hardware Subpanels.vi"() -> ()  [unwired: 12 in]
  n451 = vi-ref "RxnRover.lvlib:Hardware Subpanels.vi"() -> (w41:refnum<vi>)
  n452 = invoke on="Reactor Status Indicators" class="SubPnl" method="Insert VI"("VI Ref"=w41) -> ()  [unwired: 3 in, 4 out]
  n453 = Unregister For Events(event registration refnum=w32) -> (error out=w6:errorcluster)  [unwired: 1 in]
  n454 = Destroy User Event(user event=w10, error in=w6) -> (error out=w31:errorcluster)
  n455 = Destroy User Event(user event=w33, error in=w6) -> (error out=w30:errorcluster)
  n456 = Destroy User Event(user event=w27, error in=w6) -> (error out=w26:errorcluster)
  n457 = Destroy User Event(user event=w34, error in=w6) -> (error out=w22:errorcluster)
  n458 = Destroy User Event(user event=w25, error in=w6) -> (error out=w21:errorcluster)
  n459 = Destroy User Event(user event=w23, error in=w6) -> (error out=w20:errorcluster)
  n460 = Destroy User Event(user event=w24, error in=w6) -> (error out=w18:errorcluster)
  n461 = Destroy User Event(user event=w19, error in=w6) -> (error out=w17:errorcluster)
  n462 = Destroy User Event(user event=w9, error in=w6) -> (error out=w5:errorcluster)
  n463 = Destroy User Event(user event=w8, error in=w6) -> (error out=w4:errorcluster)
  n464 = Destroy User Event(user event=w7, error in=w6) -> (error out=w3:errorcluster)
  n465 = Merge Errors(w31, w30, w26, w22, w21, w20, w18, w17, w5, w4, w3) -> (w29:errorcluster)
  n466 = Merge Errors(w42, w29) -> (w11:errorcluster)
  n467 = disable-structure shown="Default" {
    disable-tunnel: w11 -> [w920 _]
    frame condition #0 (active) {
      n468 = call <vilib>:"Simple Error Handler.vi"("error in (no error)"=w920) -> ()  [unwired: 4 in, 5 out]
    }
    frame condition #1 {
      # "Call Quit LabVIEW if running as a built application."
      n469 = Quit LabVIEW() -> ()  [unwired: 1 in]
    }
  }
